vi "GIS Poll Process.vi"(8 "error in (no error)":errorcluster, 9 "notifierSync":refnum<notifier>, 10 "TopLevel":refnum<class "TopLevel.lvclass">, 11 "GIS Printer in":refnum<class "GIS Printer.lvclass">) -> (0 "error out":errorcluster, 3 "GIS Printer out":refnum<class "GIS Printer.lvclass">)   [LabVIEW 2022 SP3, in "GIS Printer.lvclass"]
uses:
  GIS Printer.lvclass
  TopLevel/TopLevel.lvclass
  GIS Printer.lvclass/GIS Printer.ctl
  Typedefs/GIS_PollTimers--cluster.ctl
  Methods/Variant_To_DVR.vi
  Methods/Generate PollStatus Event GIS Printer.vi
panel:
  in  "C1":bool
  in  "A1":bool
  in  "C2":bool
  in  "A2":bool
  in  "C3":bool
  in  "A3":bool
  in  "C4":bool
  in  "A4":bool
  in  "C33":bool
  in  "I33 3":bool
  in  "I33 2":bool
  in  "I33 1":bool
  in  "A33":bool
  in  "C22":bool
  in  "A22":bool
  in  "C11":bool
  in  "A11":bool
  in  "OK":bool
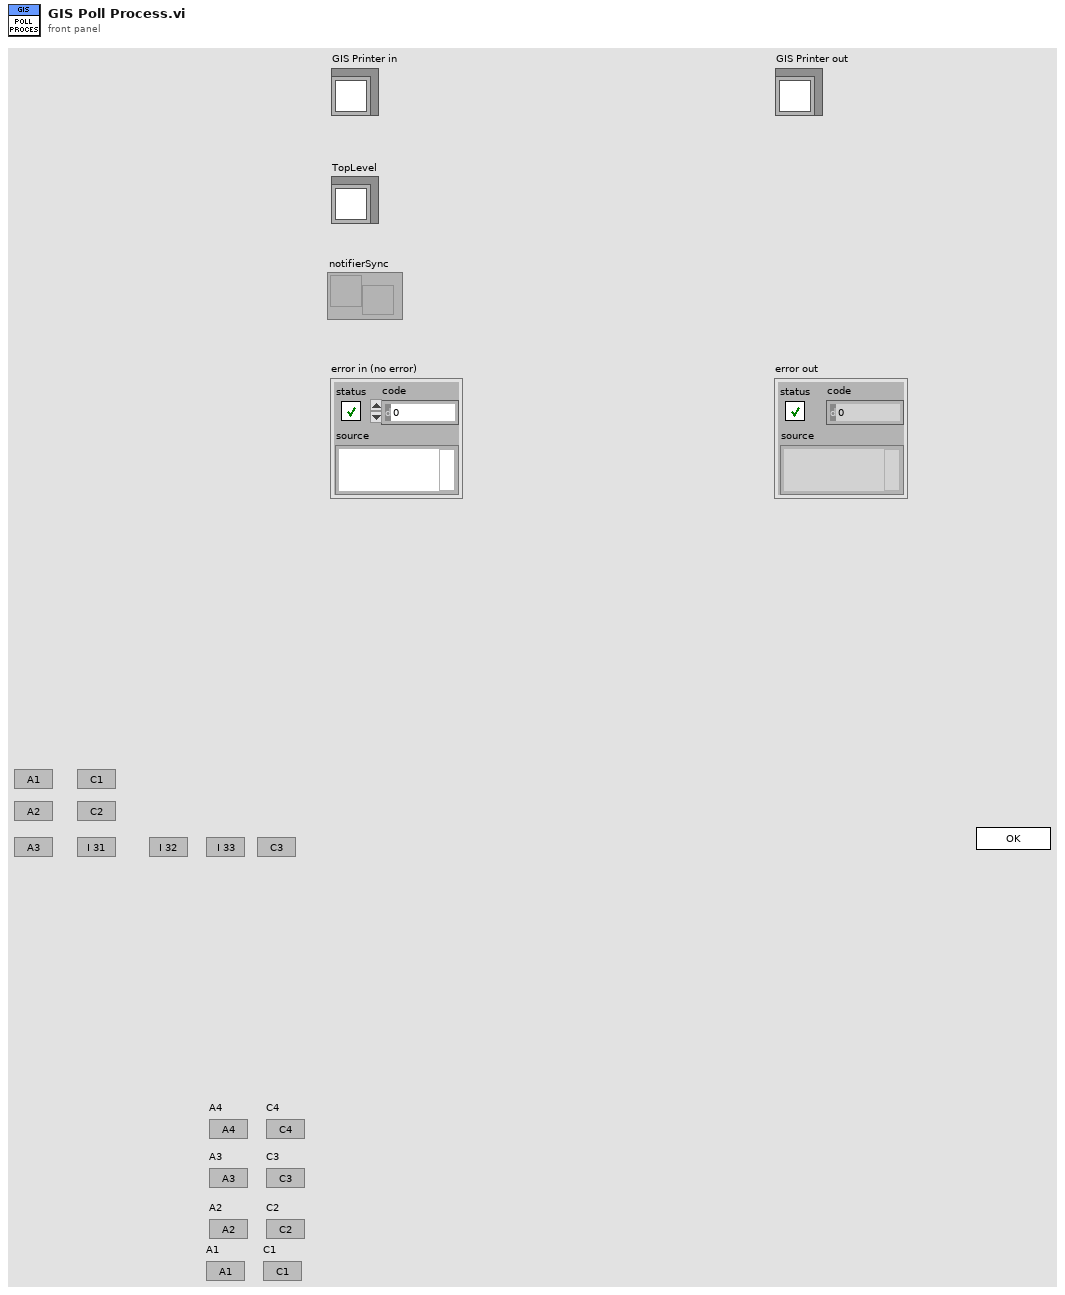
[diagram p1: front panel]
types:
  T1 = cluster{"String":string, "PrinterPollResponse":refnum<user-event>, "Open":bool, "TCP":refnum<k5>}
  T2 = enum32{"Invalid", "Standard", "Closed", "Hidden", "Minimized", "Maximized"}
  T3 = enum32{"invalid app kind", "Development System", "Run Time System", "Student Edition", "Embedded LabVIEW", "Evaluation", "Custom"}
  T4 = typedef "GIS Status--Cluster.ctl" = cluster{"HeadEnabled":bool, "SpitEnabled":bool, "HeaterEnabled":bool, "TargetTemperature":dbl, "CurrentTemperature":dbl}
  T5 = typedef "GIS Printer.lvclass/PrinterConfiguration--Cluster.ctl" = cluster{"IPAddress":string, "Move Stage on RTP Command?":bool, "Stage Move Position":string, "PH1-Prime Path":path, "PH2-Prime Path":path, "PH3-Prime Path":path, "PH4-Prime Path":path, "PH5-Prime Path":path, "PH6-Prime Path":path, "PrintScriptsFolder":path, "PurgeScriptsFolder":path, "StageScriptsFolder":path, "PH1-HeatOn Path":path, "PH2-HeatOn Path":path, "PH3-HeatOn Path":path, "PH4-HeatOn Path":path, "PH5-HeatOn Path":path, "PH6-HeatOn Path":path, "PH1-HeatOff Path":path, "PH2-HeatOff Path":path, "PH3-HeatOff Path":path, "PH4-HeatOff Path":path, "PH5-HeatOff Path":path, "PH6-HeatOff Path":path}
  T6 = typedef "GIS_PollTimers--cluster.ctl" = cluster{"HeadStatus":dbl}
  T7 = cluster{"GIS Printer in":refnum<class "GIS Printer.lvclass">, "Core":cluster{"Current VI Reference":refnum<vi>, "Close Panel on Exit?":bool}, "PrinterConfiguration":T5, "TCP":refnum<k5>, "PollTimers":T6, "PollTracker":cluster{"HeadStatusPollStart":dbl, "Poll":bool}, "notifierSync":refnum<notifier>, "PollEnable":bool}
  T8 = cluster{"Current VI Reference":refnum<vi>, "Close Panel on Exit?":bool}
  T9 = typedef "TopLevel.lvclass/Digilens Config Cluster.ctl" = cluster{"Motion Controller":T10, "IO Config":T11, "PrinterConfiguration":T5, "DAQ Settings":T14}
  T10 = typedef "Motor Controller.lvclass/Motor Controller Config Data.ctl" = cluster{"Motor IP Addresss":string, "Current Position":i32, "Pulse_Per_mm":i32, "PrePrint":dbl[], "Load Position_mm":i32, "Laminate Position_mm":i32}
  T11 = typedef "IO.lvclass/IO Config Data.ctl" = cluster{"DAQDevices":T12[], "DI Channels":T13[], "DO Channels":T13[], "Material Names":string[], "AI Channels":T13[], "AO Channels":T13[]}
  T12 = typedef "IO.lvclass/DCON_DeviceConfig--Cluster.ctl" = cluster{"COM":string, "DeviceName":string, "BaudRate":u32, "Number of Channels":i32, "DeviceAddress":i32, "Enable":bool}
  T13 = typedef "IO.lvclass/Channel Data.ctl" = cluster{"Channel Name":string, "Device Name":string, "Channel No":string}
  T14 = typedef "DAQ.lvclass/TD DAQ Settings--cluster.ctl" = cluster{"Simulate DAQ":bool, "DI Settings":T15[], "AI Settings":T16[], "Relay IONames":string[], "AO IONames":string[], "AO NChan SingleTask":bool}
  T15 = typedef "DAQ.lvclass/TD DI Instrument Settings--cluster.ctl" = cluster{"Disable":bool, "DI TaskName":string, "DI RefreshIntv":i32}
  T16 = typedef "DAQ.lvclass/TD AI Instrument Settings--cluster.ctl" = cluster{"Disable":bool, "AI TaskName":string, "AI InstSettings":T17, "SimAI Ranges":T18}
  T17 = typedef "DAQ.lvclass/TD AI InstSettings--cluster.ctl" = cluster{"DaqRate":dbl, "NumSamples":i32}
  T18 = typedef "DAQ.lvclass/TD SimAI Ranges--cluster.ctl" = cluster{"lo":dbl, "hi":dbl}
  T19 = typedef "TopLevel.lvclass/UserEvents.ctl" = cluster{"API Incoming Event":refnum<user-event>, "API Executed Event":refnum<user-event>, "API Return Event":refnum<user-event>, "Exit Event":refnum<user-event>, "StatusChanged":refnum<user-event>, "DLP GUI Config Changed":refnum<user-event>, "AppEvent":refnum<user-event>, "Login Event":refnum<user-event>}
  T20 = typedef "GIS Printer.lvclass/UserEvents.ctl" = cluster{"API Incoming Event":refnum<user-event>, "API Executed Event":refnum<user-event>, "API Return Event":refnum<user-event>, "Status Changed Event":refnum<user-event>, "Abort":refnum<user-event>, "stop process":refnum<user-event>, "GISPollStatus":refnum<user-event>, "GISHeadStatus":refnum<user-event>, "Error Event":refnum<user-event>}
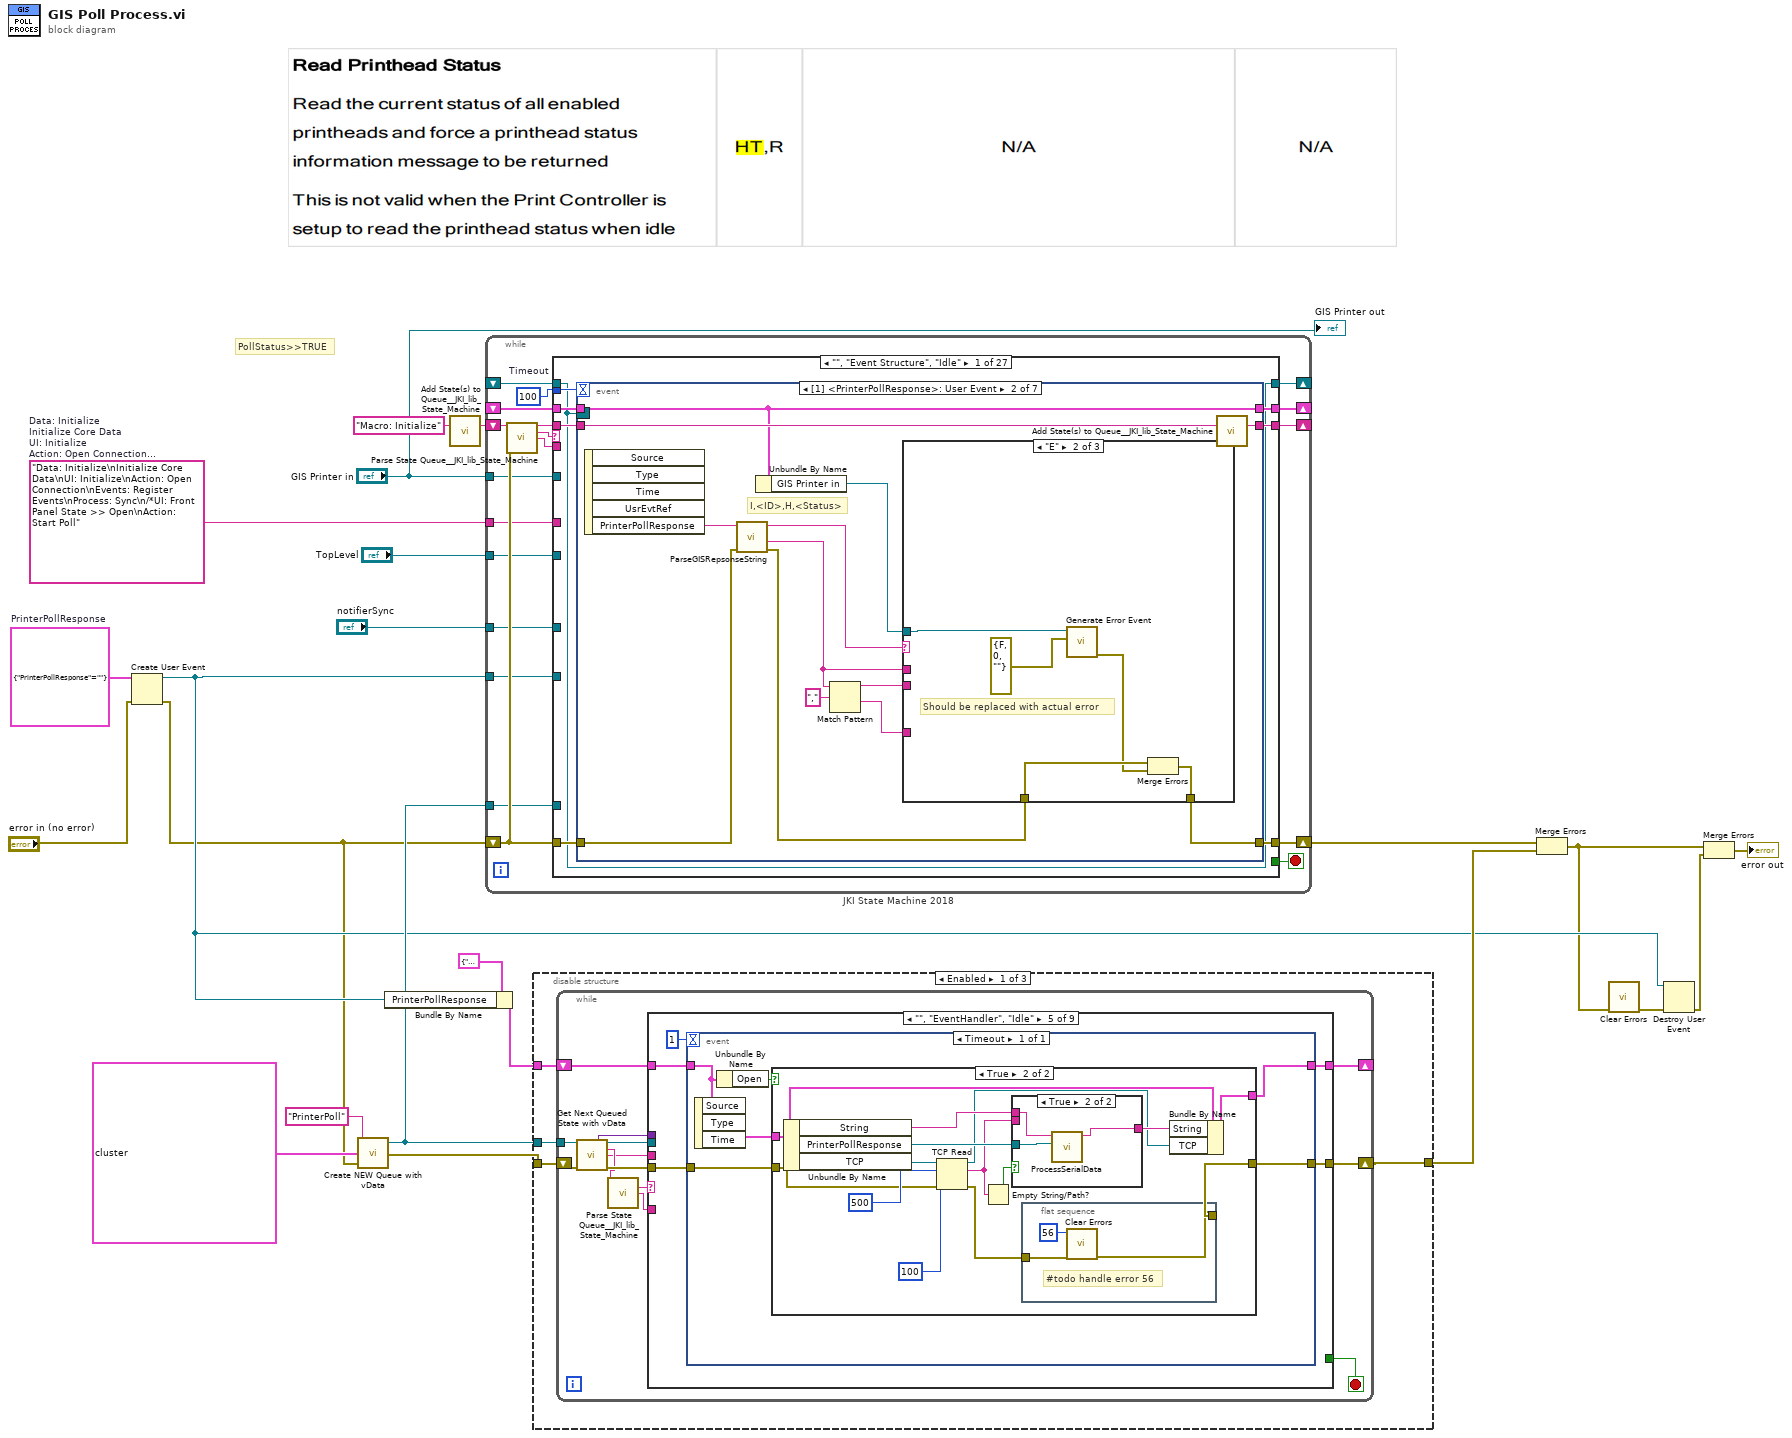
[diagram p0: block diagram]
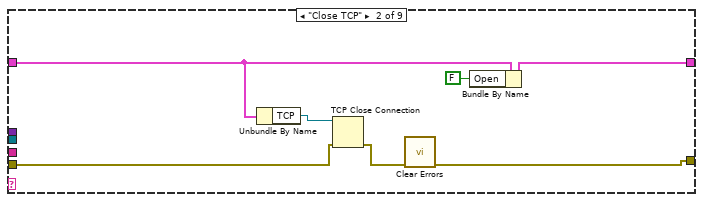
[diagram p3: hidden frame]
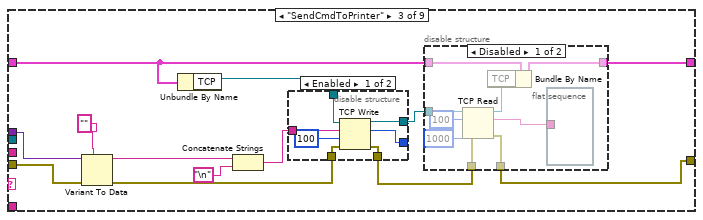
[diagram p4: hidden frame]
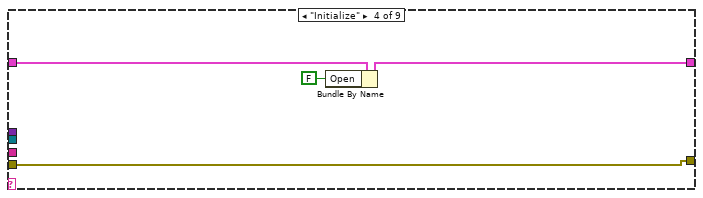
[diagram p7: hidden frame]
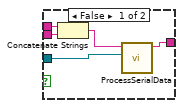
[diagram p9: hidden frame]
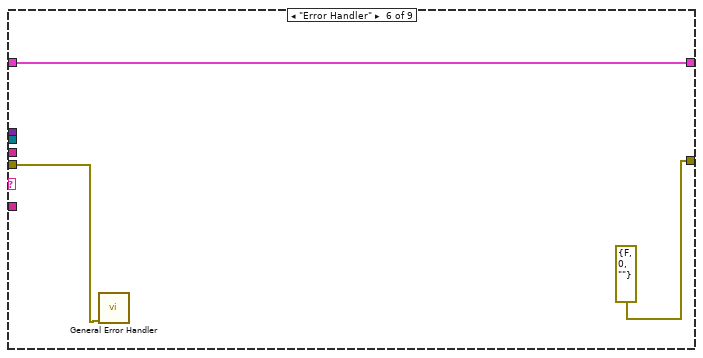
[diagram p10: hidden frame]
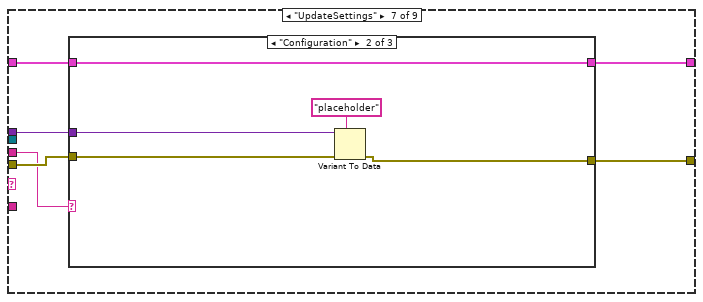
[diagram p11: hidden frame]
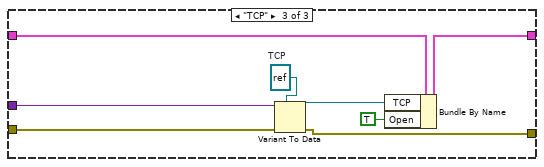
[diagram p13: hidden frame]
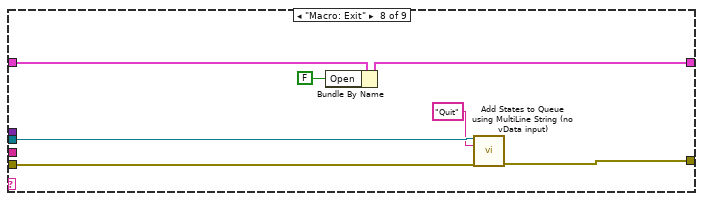
[diagram p14: hidden frame]
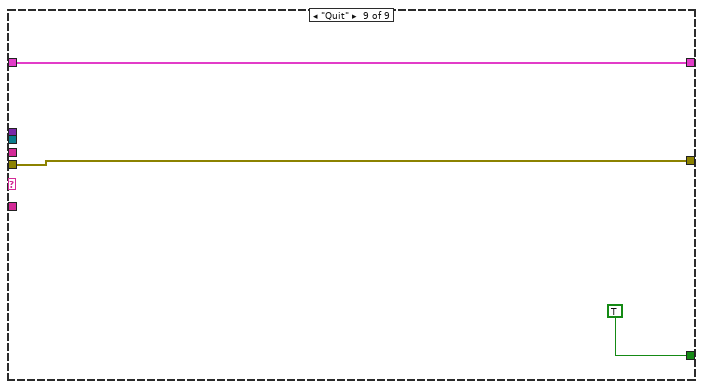
[diagram p15: hidden frame]
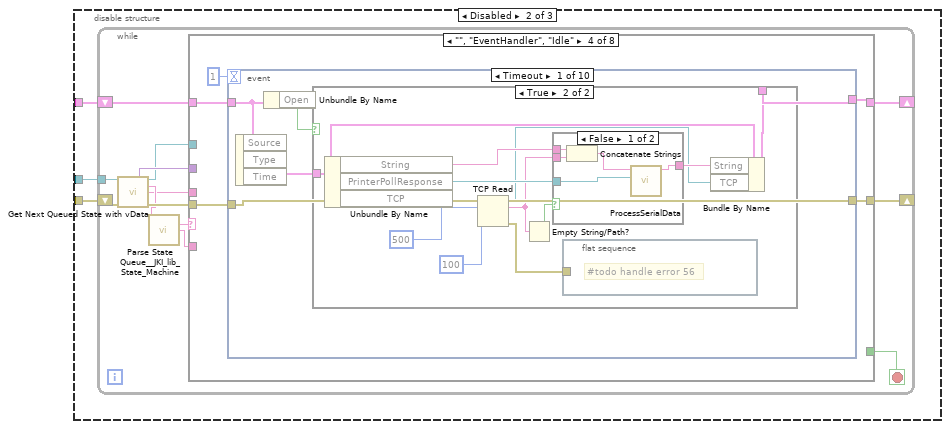
[diagram p16: hidden frame]
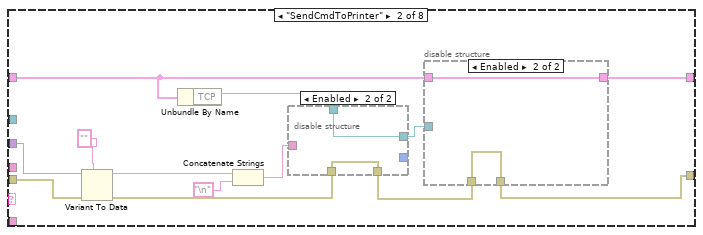
[diagram p18: hidden frame]
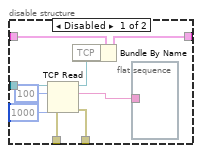
[diagram p19: hidden frame]
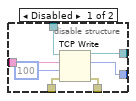
[diagram p20: hidden frame]
diagram:
  w1 = "Data: Initialize\nInitialize Core Data\nUI: Initialize\nAction: Open Connection\nEvents: Register Events\nProcess: Sync\n/*UI: Front Panel State >> Open\nAction: Start Poll"  # Data: Initialize Initialize Core Data UI: Initialize Action: Open Connection Events: Register Events Process: Sync /*UI: Front Panel State >> Open Action: Start Poll
  w13 = cluster{"PrinterPollResponse":string} {"PrinterPollResponse"=""}  # PrinterPollResponse
  # "PollStatus>>TRUE"
  n1 = Create User Event(user event datatype=w13, error in="error in (no error)") -> (user event=w10:refnum<user-event>, error out=w2:errorcluster)
  n2 = call <vilib>:"Create NEW Queue with vData.vi"("error in (no error)"=w2, "Initial States"=cluster{"state":string, "vData":variant}[] [{"state"="Initialize", "vData"=variant}, {"state"="Idle", "vData"=variant}], "Name (SMQ)"="PrinterPoll") -> ("error out"=w18:errorcluster, "queue out"=w14:refnum<queue>)  [unwired: 1 in]
  n3 = Bundle By Name(cluster=T1 {"String"="", "PrinterPollResponse"=refnum, "Open"=FALSE, "TCP"=refnum}, "PrinterPollResponse"=w10) -> (w15:T1)
  n4 = call <vilib>:"Add State(s) to Queue__JKI_lib_State_Machine.vi"("State(s) in (\"\")"="Macro: Initialize") -> ("States Out"=w22:string)  [unwired: 14 in]
  n5 = while "JKI State Machine 2018" {
    shift-right: [w34] -> _
    shift-left: _ -> [w33]
    shift-right: [w37] -> w12
    shift-left: w2 -> [w31]
    shift-right: [w36] -> _
    shift-left: w22 -> [w38]
    tunnel: "GIS Printer in" -> [w30]
    tunnel: "TopLevel" -> [w29]
    tunnel: w14 -> [w28]
    tunnel: w10 -> [w27]
    shift-right: [w26] -> _
    shift-left: _ -> [w25]
    tunnel: "notifierSync" -> [w24]
    tunnel: w1 -> [w23]
    stop <- w35 stop-if-true
    w32 = 100  # Timeout
    n6 = call <vilib>:"Parse State Queue__JKI_lib_State_Machine.vi"("State Queue"=w38, "Error In (no error)"=w31) -> ("Remaining States"=w40:string, "Current State"=w41:string, "Arguments"=w39:string)  [unwired: 11 in]
    n7 = case shown="\"\", \"Event Structure\", \"Idle\"" w41 {
      selector: w41 -> [_ _ w136 _ _ _ _ _ _ _ _ _ _ _ _ _ _ _ _ _ _ _ _ _ _ _ _]
      tunnel: w40 -> [w49 w134 w140 w160 w167 w176 w181 w188 w202 w217 w224 w229 w234 w241 w253 w323 w329 w340 w345 w353 w361 w375 w384 w399 w405 w417 w428]
      tunnel: w39 -> [_ _ _ _ _ _ _ _ _ _ _ _ _ w236 w247 _ _ _ _ _ _ _ _ _ _ w413 _]
      tunnel: w33 -> [w47 w131 w138 w153 w164 w174 w178 w186 w195 _ w219 w226 w232 w239 w249 w320 w326 w337 w342 w350 w356 w371 w381 w394 w403 w415 w418]
      tunnel: [w46 w132 w142 w157 errorcluster {"status"=FALSE, "code"=0, "source"=""} ("error out") w169 w179 w184 w191 w203 w220 w227 w231 w237 w250 w321 w327 w338 w343 w347 w355 w373 w382 w390 w401 w411 w421] -> w37
      tunnel: w31 -> [w45 w132 w141 w157 w163 w168 w179 w183 w197 w203 w221 w227 w231 w238 w251 w321 w327 w338 w343 w346 w354 w373 w382 w386 w400 w410 w420]
      tunnel: [w48 w133 w139 w159 w166 w175 w180 w187 w201 w216 w223 w228 w233 w240 w252 w322 w328 w339 w344 w352 w360 w374 w383 w398 w404 w416 w427] -> w36
      tunnel: [_ _ _ _ _ TRUE _ _ _ _ _ _ _ _ _ _ _ _ _ _ _ _ _ _ _ _ _] -> w35
      tunnel: [w44 w131 w138 w158 w164 w174 w178 w186 w196 w215 w219 w226 w232 w239 w249 w320 w326 w337 w342 w350 w356 w371 w379 w394 w403 w408 w419] -> w34
      tunnel: w32 -> [w43 _ _ _ _ _ _ _ _ _ _ _ _ _ _ _ _ _ _ _ _ _ _ _ _ _ _]
      tunnel: w30 -> [_ _ _ _ _ _ _ _ _ w204 _ _ _ _ _ _ _ _ _ _ _ _ _ _ _ _ _]
      tunnel: w29 -> [_ _ _ _ _ _ _ _ _ w213 _ _ _ _ _ _ _ _ _ _ _ _ _ w388 _ _ _]
      tunnel: w28 -> [_ _ _ _ _ w170 _ _ w193 _ _ _ _ _ _ _ _ _ _ w348 _ _ _ _ _ w412 w422]
      tunnel: w27 -> [_ _ _ _ _ _ _ _ _ _ _ _ _ _ _ _ _ _ _ _ _ _ _ w397 _ _ _]
      tunnel: [w42 w130 w135 w147 w161 w172 w177 w182 w189 w209 w218 w225 w230 w235 w246 w319 w325 w330 w341 w351 w359 w372 w380 w396 w402 w409 w426] -> w26
      tunnel: w25 -> [w42 w130 w135 w147 w161 w172 w177 w182 w189 w209 w218 w225 w230 w235 w246 w319 w325 w330 w341 w351 w359 w372 w380 _ w402 w409 w426]
      tunnel: w24 -> [_ _ _ _ _ _ _ _ _ w206 _ _ _ _ _ _ _ _ _ _ _ _ _ _ _ _ _]
      tunnel: w23 -> [_ _ _ _ _ _ _ _ _ _ _ _ _ _ _ _ w324 _ _ _ _ _ _ _ _ _ _]
      frame "", "Event Structure", "Idle" {
        n8 = event shown="[1] <PrinterPollResponse>: User Event" {
          selector: w42 -> [_ _ _ _ _ _ _]
          dyn-events: _ -> [_ _ _ _ _ _ _]
          timeout: w43 -> [_ _ _ _ _ _ _]
          tunnel: w49 -> [w57 w71 w97 w102 w106 w114 w129]
          tunnel: [w56 w70 w96 w101 w105 w113 w128] -> w48
          tunnel: w47 -> [w53 w63 w94 w99 w103 w109 w126]
          tunnel: [w55 w61 w95 w100 w104 w108 w127] -> w46
          tunnel: w45 -> [w55 w59 w95 w100 w104 w107 w127]
          tunnel: [w53 w63 w94 w99 w103 w110 w126] -> w44
          event Timeout {
            n9 = event-data() -> ()  [unwired: 1 in, 1 out]
            n10 = Unbundle By Name(w53) -> ("PollTracker.Poll"=w52:bool, "PollEnable"=w50:bool)
            n11 = And(x=w52, y=w50) -> (x .and. y?=w51:bool)
            n12 = case shown="True" w51 {
              tunnel: [_ "Action: CheckPollTimers" ("State(s) in Front (\"\")")] -> w54
              frame False {
              }
              frame True {
              }
            }
            n13 = call <vilib>:"Add State(s) to Queue__JKI_lib_State_Machine.vi"("State(s) in Front (\"\")"=w54, "State(s) in (\"\")"=w57) -> ("States Out"=w56:string)  [unwired: 13 in]
          }
          event User Event {
            # "I,<ID>,H,<Status>"
            n14 = event-data() -> ("PrinterPollResponse"=w69:string)  [unwired: 1 in, 4 out]
            n15 = call "ParseGISRepsonseString.vi"("error in (no error)"=w59, "Response In"=w69) -> ("error out"=w60:errorcluster, "Status"=w66:string, "Category"=w68:string)  [unwired: 6 in, 1 out]
            n16 = Unbundle By Name(w63) -> ("GIS Printer in"=w62:refnum<class "GIS Printer.lvclass">)
            n17 = Match Pattern(string=w66, regular expression=",") -> (before substring=w65:string, after substring=w64:string)  [unwired: 1 in, 2 out]
            n18 = case shown="\"E\"" w68 {
              tunnel: w66 -> [_ _ _]
              tunnel: w65 -> [_ _ w84]
              tunnel: w64 -> [_ _ w81]
              tunnel: w62 -> [_ w77 w80]
              tunnel: w60 -> [w72 w75 w79]
              tunnel: [w72 w73 w78] -> w61
              frame Default {
              }
              frame "E" {
                # "Should be replaced with actual error"
                n19 = call-dynamic "Generate Error Event.vi"("Error"=errorcluster {"status"=FALSE, "code"=0, "source"=""}, "GIS Printer in"=w77) -> ("error out"=w74:errorcluster)  [unwired: 8 in, 1 out]
                n20 = Merge Errors(w75, w74) -> (w73:errorcluster)
              }
              frame "I" {
                n21 = Equal?(x=w84, y="H") -> (x = y?=w82:bool)
                n22 = case shown="True" w82 {
                  tunnel: w81 -> [_ w92]
                  tunnel: w80 -> [_ w90]
                  tunnel: w79 -> [w85 w91]
                  tunnel: [w85 w87] -> w78
                  frame False {
                  }
                  frame True {
                    n23 = call "GISStatus_XML_Read.vi"("error in (no error)"=w91, "XML String"=w92) -> ("error out"=w88:errorcluster, "HeadStatus"=w89:T4[])  [unwired: 7 in, 1 out]
                    n24 = call "Write GISPollStatus.vi"("ForceEvent"=TRUE, "error in (no error)"=w88, "GISHeadStatus"=w89, "GIS Printer in"=w90) -> ("error out"=w87:errorcluster)  [unwired: 6 in, 1 out]
                  }
                }
              }
            }
            n25 = call <vilib>:"Add State(s) to Queue__JKI_lib_State_Machine.vi"("State(s) in (\"\")"=w71) -> ("States Out"=w70:string)  [unwired: 14 in]
          }
          event "OK": Value Change {
            # "Exit Button Value Change (pressed) Event\n(this executes Macro: Exit to terminate the VI)"
            n26 = event-data() -> ()  [unwired: 1 in, 1 out]
            n27 = call <vilib>:"Add State(s) to Queue__JKI_lib_State_Machine.vi"("State(s) in Front (\"\")"="Macro: Exit", "State(s) in (\"\")"=w97) -> ("States Out"=w96:string)  [unwired: 13 in]
          }
          event User Event {
            # "Exit Button Value Change (pressed) Event\n(this executes Macro: Exit to terminate the VI)"
            n28 = event-data() -> ()  [unwired: 1 in, 5 out]
            n29 = call <vilib>:"Add State(s) to Queue__JKI_lib_State_Machine.vi"("State(s) in Front (\"\")"="Macro: Exit", "State(s) in (\"\")"=w102) -> ("States Out"=w101:string)  [unwired: 13 in]
          }
          event User Event {
            # "#TODO API: Abort called in  other process. do something about it man!\njust do something...anything"
            # "Exit Button Value Change (pressed) Event\n(this executes Macro: Exit to terminate the VI)"
            n30 = event-data() -> ()  [unwired: 1 in, 5 out]
            n31 = call <vilib>:"Add State(s) to Queue__JKI_lib_State_Machine.vi"("State(s) in (\"\")"=w106) -> ("States Out"=w105:string)  [unwired: 14 in]
          }
          event User Event {
            n32 = event-data() -> ("Command"=w112:string, "Data"=w111:variant)  [unwired: 1 in, 4 out]
            n33 = case shown="\"StatusPoll\"" w112 {
              tunnel: w111 -> [_ w123]
              tunnel: w109 -> [w116 w121]
              tunnel: [w116 w120] -> w110
              tunnel: w107 -> [w115 w118]
              tunnel: [w115 w117] -> w108
              frame Default {
              }
              frame "StatusPoll" {
                n34 = Variant To Data(error in=w118, type=FALSE, Variant=w123) -> (data=w119:bool, error out=w117:errorcluster)
                n35 = Bundle By Name(cluster=w121, "PollEnable"=w119) -> (w120:T7)
              }
            }
            n36 = call <vilib>:"Add State(s) to Queue__JKI_lib_State_Machine.vi"("State(s) in (\"\")"=w114) -> ("States Out"=w113:string)  [unwired: 14 in]
          }
          event Panel Close? {
            # "Discard the event because we'll close the front panel ourselves in Macro: Exit"
            # "Close Panel button (pressed) Event\n(this executes Macro: Exit to terminate the VI)"
            n37 = event-data() -> ()  [unwired: 1 in, 1 out]
            n38 = event-data("Discard?"=TRUE) -> ()  [unwired: 1 in, 1 out]
            n39 = call <vilib>:"Add State(s) to Queue__JKI_lib_State_Machine.vi"("State(s) in Front (\"\")"="Macro: Exit", "State(s) in (\"\")"=w129) -> ("States Out"=w128:string)  [unwired: 13 in]
          }
        }
      }
      frame "---------- Core ----------" {
        # "Do not put any code in this frame.\n(it is a separator no-op)"
        n40 = call <vilib>:"Add State(s) to Queue__JKI_lib_State_Machine.vi"("State(s) in (\"\")"=w134) -> ("States Out"=w133:string)  [unwired: 14 in]
      }
      frame Default {
        w145 = 42 items=["No error", "Argument error", "Memory is full", "Out of zone", "End of file", "File already open", "Generic file I/O error", "File not found", "File permission error", "Disk is full", "Duplicate path", "Too many files open", "System feature not enabled", "Resource file not found", "Cannot add resource", "Resource not found", "Image not found", "Image memory error", "Pen does not exist", "Config type invalid", "Config token not found", "Config parse error", "Config memory error", "Bad external code format", "Bad external code offset", "External code not present", "Null window", "Destroy window error", "Null menu", "Print aborted", "Bad print record", "Print driver error", "Windows error during printing", "Memory error during printing", "Print dialog error", "Generic print error", "Invalid device refnum", "Device not found", "Device parameter error", "Device unit error", "Cannot open device", "Device call aborted", "Generic error", "Cancelled by user", "Object ID too low", "Object ID too high", "Object not in heap", "Unknown heap", "Unknown object (invalid DefProc)", "Unknown object (DefProc not in table)", "Message out of range", "Invalid (null) method", "Unknown message", "Manager call not supported", "Bad address", "Network operation in progress", "Network operation timed out", "Connection is busy", "Network attribute not supported", "Network error", "Address in use", "System out of memory", "Connection aborted", "Connection refused", "Not connected", "Already connected", "Connection closed", "Initialization error (interapplication manager)", "Bad occurrence", "Wait on unbound occurrence handler", "Occurrence queue overflow", "Datalog type conflict", "Unused", "Unrecognized type (interapplication manager)", "Memory corrupt", "Failed to make temporary DLL", "Old CIN version", "Drag socket not found", "Failed to load drop-object", "Failed to register OLE object", "Failed to release OLE object", "Format specifier type mismatch", "Unknown format specifier", "Too few format specifiers", "Too many format specifiers", "Scan failed", "Newer CIN version", "Error converting to variant", "Runtime menu error", "Password tampered", "Variant attribute not found", "Incompatible variant data type", "Event data is not available", "Event Store is not present", "Occurrence is not found", "Event Queue is not created", "Event info is not available", "Refnum passed is NULL", "Error retrieving Class GUID", "Error retrieving CoClass GUID", "Error retrieving TypeLib GUID.", "Bad built application magic bytes.", "Specific driver is different from the specific driver associated with the Logical Name.", "There is no session opened to the class driver.", "Max Error", "MAX - Error with config objects", "MAX - Error loading configuration", "MAX - Group not supported"]
        # "Current State"
        # "Do not delete, rename, or modify this frame.\n(this is used to capture unhandled states and typos)"
        # "Handle mistyped state name (developer tool)"
        n41 = Format Into String(format string="Software Exception: Unhandled State \"%s\"." ("message"), error in=w141, w136) -> (resulting string=w144:string, error out=w143:errorcluster)  [unwired: 1 in]
        n42 = call <vilib>:"Error Cluster From Error Code.vi"("show call chain? (False)"=TRUE, "error in (no error)"=w143, "error message (\"\")"=w144, "error code (0)"=w145) -> ("error out"=w142:errorcluster)  [unwired: 5 in]
        n43 = call <vilib>:"Add State(s) to Queue__JKI_lib_State_Machine.vi"("State(s) in (\"\")"=w140) -> ("States Out"=w139:string)  [unwired: 14 in]
      }
      frame "Initialize Core Data" {
        # "Do not delete, rename, or modify this frame.\n(this is used to determine panel behavior on exit)"
        # "originally closed?"
        # "exe?"
        # "If panel starts closed or is an EXE, then close it when we exit"
        n44 = property class="VI"() -> ("FP.State"=w150:T2)  [unwired: 2 in, 2 out]
        n45 = property class="App"() -> ("App.Kind"=w156:T3)  [unwired: 2 in, 2 out]
        n46 = control-ref of="Current VI Reference"() -> (w151:refnum<vi>)
        n47 = Equal?(x=w150, y=T2."Closed" ("Front Panel Window:State")) -> (x = y?=w148:bool)
        n48 = Equal?(x=w156, y=T3."Run Time System" ("Application:Kind")) -> (x = y?=w154:bool)
        n49 = Or(x=w148, y=w154) -> (x .or. y?=w152:bool)
        n50 = Bundle By Name(cluster=w153, "Core.Current VI Reference"=w151, "Core.Close Panel on Exit?"=w152) -> (w158:T7)
        n51 = call <vilib>:"Add State(s) to Queue__JKI_lib_State_Machine.vi"("State(s) in (\"\")"=w160) -> ("States Out"=w159:string)  [unwired: 14 in]
      }
      frame "Error Handler" {
        # "Unhandled Error -- Display it"
        # "Handle any errors here.\nYou can also output any states to clean-up after errors occur"
        # "Clear error"
        n52 = call <vilib>:"General Error Handler.vi"("error in (no error)"=w163) -> ()  [unwired: 10 in, 5 out]
        n53 = call <vilib>:"Add State(s) to Queue__JKI_lib_State_Machine.vi"("State(s) in Front (\"\")"="/* Post Error States", "State(s) in (\"\")"=w167) -> ("States Out"=w166:string)  [unwired: 13 in]
      }
      frame "Exit" {
        n54 = call <vilib>:"Add States to Queue using MultiLine String (no vData input).vi"("queue in"=w170, "states in"="Quit", "error in"=w168) -> ("error out"=w169:errorcluster)  [unwired: 10 in, 2 out]
        n55 = call <vilib>:"Add State(s) to Queue__JKI_lib_State_Machine.vi"("State(s) in (\"\")"=w176) -> ("States Out"=w175:string)  [unwired: 14 in]
      }
      frame "---------- Data ----------" {
        # "Do not put any code in this frame.\n(It is a separator no-op. You can make a copy of this frame to create a new Data frame)"
        n56 = call <vilib>:"Add State(s) to Queue__JKI_lib_State_Machine.vi"("State(s) in (\"\")"=w181) -> ("States Out"=w180:string)  [unwired: 14 in]
      }
      frame "Data: GIS Disconnect" {
        # "Do not put any code in this frame.\n(It is a separator no-op. You can make a copy of this frame to create a new Data frame)"
        n57 = Unbundle By Name(w186) -> ("TCP"=w185:refnum<k5>)
        n58 = TCP Close Connection(connection ID=w185, error in (no error)=w183) -> (error out=w184:errorcluster)  [unwired: 1 in, 1 out]
        n59 = call <vilib>:"Add State(s) to Queue__JKI_lib_State_Machine.vi"("State(s) in (\"\")"=w188) -> ("States Out"=w187:string)  [unwired: 14 in]
      }
      frame "Data: GIS Connect" {
        n60 = Unbundle By Name(w195) -> ("PrinterConfiguration.IPAddress"=w200:string)
        n61 = TCP Open Connection(address=w200, remote port or service name=u16 2000, timeout ms (60000)=1000, error in (no error)=w197) -> (connection ID=w190:refnum<k5>, error out=w192:errorcluster)  [unwired: 1 in]
        n62 = call <vilib>:"Add State to Queue with vData.vi"("queue in"=w193, "state in"="UpdateSettings>>TCP", "vData (\"\")"=w190, "error in"=w192) -> ("error out"=w191:errorcluster)  [unwired: 8 in, 3 out]
        n63 = Bundle By Name(cluster=w195, "TCP"=w190) -> (w196:T7)
        n64 = call <vilib>:"Add State(s) to Queue__JKI_lib_State_Machine.vi"("State(s) in (\"\")"=w202) -> ("States Out"=w201:string)  [unwired: 14 in]
      }
      frame "Data: Initialize" {
        w205 = TRUE  # PollEnable
        w207 = cluster{"HeadStatusPollStart":dbl, "Poll":bool} {"HeadStatusPollStart"=0.0, "Poll"=FALSE}  # PollTracker
        w208 = T6 {"HeadStatus"=2.0}  # PollTimers
        w210 = refnum<k5> refnum  # TCP
        w214 = T8 {"Current VI Reference"=refnum, "Close Panel on Exit?"=FALSE}  # Core
        # "#TODO get from config"
        n65 = property class="TopLevel.lvclass"(reference=w213) -> ("Methods:Accessors:Digilens Config"=w212:T9)  [unwired: 1 in, 2 out]
        n66 = Unbundle By Name(w212) -> ("PrinterConfiguration"=w211:T5)
        n67 = Bundle("GIS Printer in"=w204, "Core"=w214, "PrinterConfiguration"=w211, "TCP"=w210, "PollTimers"=w208, "PollTracker"=w207, "notifierSync"=w206, "PollEnable"=w205) -> (w215:T7)  [unwired: 1 in]
        n68 = call <vilib>:"Add State(s) to Queue__JKI_lib_State_Machine.vi"("State(s) in (\"\")"=w217) -> ("States Out"=w216:string)  [unwired: 14 in]
      }
      frame "Data: Cleanup" {
        # "Cleanup any data and references, here.\n(this is called automatically, by the Macro: Exit)"
        n69 = Unbundle By Name(w219) -> ("Core.Current VI Reference"=w222:refnum<vi>)
        n70 = Close Reference(reference=w222, error in (no error)=w221) -> (error out=w220:errorcluster)
        n71 = call <vilib>:"Add State(s) to Queue__JKI_lib_State_Machine.vi"("State(s) in (\"\")"=w224) -> ("States Out"=w223:string)  [unwired: 14 in]
      }
      frame "---------- UI ----------" {
        # "Do not put any code in this frame.\n(It is a separator no-op. You can make a copy of this frame to create a new UI frame)"
        n72 = call <vilib>:"Add State(s) to Queue__JKI_lib_State_Machine.vi"("State(s) in (\"\")"=w229) -> ("States Out"=w228:string)  [unwired: 14 in]
      }
      frame "UI: Initialize" {
        n73 = call <vilib>:"Add State(s) to Queue__JKI_lib_State_Machine.vi"("State(s) in (\"\")"=w234) -> ("States Out"=w233:string)  [unwired: 14 in]
      }
      frame "UI: Cursor Set" {
        # "Argument"
        # "Set and Unset Cursor Busy.\n(Usage: \"UI: Cursor Set >> Busy|Idle\")"
        n74 = case shown="\"Idle\", Default" w236 {
          tunnel: w238 -> [w243 w245]
          tunnel: [w242 w244] -> w237
          frame "Idle", Default {
            n75 = call <vilib>:"Unset Busy.vi"("error in (no error)"=w243) -> ("error out"=w242:errorcluster)  [unwired: 10 in]
          }
          frame "Busy" {
            n76 = call <vilib>:"Set Busy.vi"("error in (no error)"=w245) -> ("error out"=w244:errorcluster)  [unwired: 9 in, 1 out]
          }
        }
        n77 = call <vilib>:"Add State(s) to Queue__JKI_lib_State_Machine.vi"("State(s) in (\"\")"=w241) -> ("States Out"=w240:string)  [unwired: 14 in]
      }
      frame "UI: Front Panel State" {
        # "Argument"
        # "Set Front Panel Open or Closed\n(Usage: \"UI: Front Panel State >> Open|Close\")"
        n78 = Unbundle By Name(w249) -> ("Core.Current VI Reference"=w248:refnum<vi>)
        n79 = case shown="\"Minimize\", \"Minimized\"" w247 {
          tunnel: w251 -> [w259 w274 w285 w298 w311]
          tunnel: [w261 w275 w287 w300 w313] -> w250
          tunnel: w248 -> [w260 w272 w286 w299 w312]
          frame "Open", "Standard", Default {
            w254 = T2."Standard" ("State")
            n80 = property class="VI"(reference=w260, error in=w259) -> (reference out=w257:refnum<vi>, error out=w258:errorcluster, "FP.State"=w256:T2)
            n81 = Not Equal?(x=w256, y=w254) -> (x != y?=w255:bool)
            n82 = case shown="True" w255 {
              tunnel: [w265 w267] -> w261
              tunnel: w258 -> [w264 w267]
              tunnel: w257 -> [w263 _]
              tunnel: w254 -> [w262 _]
              frame True {
                n83 = invoke class="VI" method="FP.Open"(reference=w263, error in=w264, "Activate"=TRUE, "State"=w262) -> (error out=w265:errorcluster)  [unwired: 1 in, 4 out]
              }
              frame False {
              }
            }
          }
          frame "Close", "Closed" {
            n84 = property class="VI"(reference=w272, error in=w274) -> (reference out=w271:refnum<vi>, error out=w273:errorcluster, "FP.State"=w269:T2)
            n85 = Not Equal?(x=w269, y=T2."Closed" ("Front Panel Window:State")) -> (x != y?=w268:bool)
            n86 = case shown="True" w268 {
              tunnel: [w276 w279] -> w275
              tunnel: w273 -> [w276 w278]
              tunnel: w271 -> [_ w277]
              frame False {
              }
              frame True {
                n87 = invoke class="VI" method="FP.Close"(reference=w277, error in=w278) -> (error out=w279:errorcluster)  [unwired: 1 in, 2 out]
              }
            }
          }
          frame "Hidden", "Hide" {
            w280 = T2."Hidden" ("State")
            n88 = property class="VI"(reference=w286, error in=w285) -> (reference out=w283:refnum<vi>, error out=w284:errorcluster, "FP.State"=w282:T2)
            n89 = Not Equal?(x=w282, y=w280) -> (x != y?=w281:bool)
            n90 = case shown="True" w281 {
              tunnel: [w291 w292] -> w287
              tunnel: w284 -> [w290 w292]
              tunnel: w283 -> [w289 _]
              tunnel: w280 -> [w288 _]
              frame True {
                n91 = invoke class="VI" method="FP.Open"(reference=w289, error in=w290, "State"=w288) -> (error out=w291:errorcluster)  [unwired: 2 in, 4 out]
              }
              frame False {
              }
            }
          }
          frame "Minimize", "Minimized" {
            w293 = T2."Minimized" ("State")
            n92 = property class="VI"(reference=w299, error in=w298) -> (reference out=w296:refnum<vi>, error out=w297:errorcluster, "FP.State"=w295:T2)
            n93 = Not Equal?(x=w295, y=w293) -> (x != y?=w294:bool)
            n94 = case shown="True" w294 {
              tunnel: [w304 w305] -> w300
              tunnel: w297 -> [w303 w305]
              tunnel: w296 -> [w302 _]
              tunnel: w293 -> [w301 _]
              frame True {
                n95 = invoke class="VI" method="FP.Open"(reference=w302, error in=w303, "State"=w301) -> (error out=w304:errorcluster)  [unwired: 2 in, 4 out]
              }
              frame False {
              }
            }
          }
          frame "Maximize", "Maximized" {
            w306 = T2."Maximized" ("State")
            n96 = property class="VI"(reference=w312, error in=w311) -> (reference out=w309:refnum<vi>, error out=w310:errorcluster, "FP.State"=w308:T2)
            n97 = Not Equal?(x=w308, y=w306) -> (x != y?=w307:bool)
            n98 = case shown="True" w307 {
              tunnel: [w317 w318] -> w313
              tunnel: w310 -> [w316 w318]
              tunnel: w309 -> [w315 _]
              tunnel: w306 -> [w314 _]
              frame True {
                n99 = invoke class="VI" method="FP.Open"(reference=w315, error in=w316, "State"=w314) -> (error out=w317:errorcluster)  [unwired: 2 in, 4 out]
              }
              frame False {
              }
            }
          }
        }
        n100 = call <vilib>:"Add State(s) to Queue__JKI_lib_State_Machine.vi"("State(s) in (\"\")"=w253) -> ("States Out"=w252:string)  [unwired: 14 in]
      }
      frame "---------- Macro ----------" {
        # "Do not put any code in this frame.\n(It is a separator no-op. You can make a copy of this frame to create a new Macro frame)"
        n101 = call <vilib>:"Add State(s) to Queue__JKI_lib_State_Machine.vi"("State(s) in (\"\")"=w323) -> ("States Out"=w322:string)  [unwired: 14 in]
      }
      frame "Macro: Initialize" {
        n102 = call <vilib>:"Add State(s) to Queue__JKI_lib_State_Machine.vi"("State(s) in Front (\"\")"=w324, "State(s) in (\"\")"=w329) -> ("States Out"=w328:string)  [unwired: 13 in]
      }
      frame "Macro: Exit" {
        n103 = Unbundle By Name(w337) -> ("Core.Close Panel on Exit?"=w336:bool)
        n104 = Select(t="UI: Front Panel State >> Close", s=w336, f="") -> (s? t:f=w333:string)
        n105 = call <vilib>:"Add State(s) to Queue__JKI_lib_State_Machine.vi"("State(s) in (\"\")"=w333, "State(s) at Back (\"\")"="Data: Cleanup\nEvents: Unregister Events\nAction: Close Connection\nExit") -> ("States Out"=w331:string)  [unwired: 13 in]
        n106 = call <vilib>:"Add State(s) to Queue__JKI_lib_State_Machine.vi"("State(s) in Front (\"\")"=w331, "State(s) in (\"\")"=w340) -> ("States Out"=w339:string)  [unwired: 13 in]
      }
      frame "----------Action----------" {
        n107 = call <vilib>:"Add State(s) to Queue__JKI_lib_State_Machine.vi"("State(s) in (\"\")"=w345) -> ("States Out"=w344:string)  [unwired: 14 in]
      }
      frame "Action: Close Connection" {
        n108 = call <vilib>:"Add States to Queue using MultiLine String (no vData input).vi"("queue in"=w348, "states in"="Close TCP", "error in"=w346) -> ("error out"=w347:errorcluster)  [unwired: 10 in, 2 out]
        n109 = call <vilib>:"Add State(s) to Queue__JKI_lib_State_Machine.vi"("State(s) in (\"\")"=w353) -> ("States Out"=w352:string)  [unwired: 14 in]
      }
      frame "Process: Sync" {
        n110 = Unbundle By Name(w356) -> ("notifierSync"=w357:refnum<notifier>)
        n111 = Send Notification(notification=TRUE, notifier=w357, error in (no error)=w354) -> (error out=w355:errorcluster)  [unwired: 1 out]
        n112 = call <vilib>:"Add State(s) to Queue__JKI_lib_State_Machine.vi"("State(s) in (\"\")"=w361) -> ("States Out"=w360:string)  [unwired: 14 in]
      }
      frame "Action: CheckPollTimers" {
        n113 = Unbundle By Name(w371) -> ("PollTracker.HeadStatusPollStart"=w368:dbl)
        n114 = Unbundle By Name(w371) -> ("PollTimers.HeadStatus"=w366:dbl)
        n115 = Get Date/Time In Seconds() -> (seconds since 1Jan1904=w370:timestamp)
        n116 = To Double Precision Float(number=w370) -> (double precision float=w369:dbl)
        n117 = Subtract(x=w369, y=w368) -> (x-y=w367:dbl)
        n118 = Greater?(x=w367, y=w366) -> (0:w362:bool)
        n119 = Select(t="Action: Send GIS Command>>P,HT,R", s=w362, f="") -> (s? t:f=w363:string)
        n120 = call <vilib>:"Add State(s) to Queue__JKI_lib_State_Machine.vi"("State(s) in Front (\"\")"=w363, "State(s) in (\"\")"=w375) -> ("States Out"=w374:string)  [unwired: 13 in]
      }
      frame "Action: Start Poll" {
        n121 = Get Date/Time In Seconds() -> (seconds since 1Jan1904=w377:timestamp)
        n122 = To Double Precision Float(number=w377) -> (double precision float=w376:dbl)
        n123 = Bundle By Name(cluster=w381, "PollTracker.Poll"=TRUE, "PollTracker.HeadStatusPollStart"=w376) -> (w379:T7)
        n124 = call <vilib>:"Add State(s) to Queue__JKI_lib_State_Machine.vi"("State(s) in (\"\")"=w384) -> ("States Out"=w383:string)  [unwired: 14 in]
      }
      frame "Events: Register Events" {
        n125 = call-dynamic "GetEvents_TopLevel.vi"("error in (no error)"=w386, "TopLevel in"=w388) -> ("error out"=w387:errorcluster, "UserEvents"=w389:T19)  [unwired: 7 in, 1 out]
        n126 = Unbundle By Name(w394) -> ("GIS Printer in"=w395:refnum<class "GIS Printer.lvclass">)
        n127 = Unbundle By Name(w389) -> ("AppEvent"=w385:refnum<user-event>)
        n128 = call-dynamic "GetEvents_GIS Printer.vi"("error in (no error)"=w387, "TopLevel in"=w395) -> ("error out"=w390:errorcluster, "UserEvents"=w393:T20)  [unwired: 7 in, 1 out]
        n129 = Unbundle By Name(w393) -> ("Abort"=w392:refnum<user-event>, "stop process"=w391:refnum<user-event>)
        n130 = register-events(w397, w392, w391, w385) -> (reference out=w396:refnum<event-registration>)  [unwired: 2 in, 1 out]
        n131 = call <vilib>:"Add State(s) to Queue__JKI_lib_State_Machine.vi"("State(s) in (\"\")"=w399) -> ("States Out"=w398:string)  [unwired: 14 in]
      }
      frame "Events: Unregister Events" {
        n132 = Unregister For Events(event registration refnum=w402, error in=w400) -> (error out=w401:errorcluster)
        n133 = call <vilib>:"Add State(s) to Queue__JKI_lib_State_Machine.vi"("State(s) in (\"\")"=w405) -> ("States Out"=w404:string)  [unwired: 14 in]
      }
      frame "Action: Send GIS Command" {
        n134 = Get Date/Time In Seconds() -> (seconds since 1Jan1904=w407:timestamp)
        n135 = To Double Precision Float(number=w407) -> (double precision float=w406:dbl)
        n136 = call <vilib>:"Add State to Queue with vData.vi"("queue in"=w412, "state in"="SendCmdToPrinter", "vData (\"\")"=w413, "error in"=w410) -> ("error out"=w411:errorcluster)  [unwired: 8 in, 3 out]
        n137 = Bundle By Name(cluster=w415, "PollTracker.HeadStatusPollStart"=w406) -> (w408:T7)
        n138 = call <vilib>:"Add State(s) to Queue__JKI_lib_State_Machine.vi"("State(s) in (\"\")"=w417) -> ("States Out"=w416:string)  [unwired: 14 in]
      }
      frame "Action: Open Connection" {
        n139 = disable-structure shown="Enabled" {
          disable-tunnel: w420 -> [w435 w436]
          disable-tunnel: w418 -> [w434 _]
          disable-tunnel: [w432 w436] -> w425
          disable-tunnel: [w431 refnum<k5> refnum ("connection ID")] -> w424
          frame Enabled {
            (unwired) "localhost" ("address")
            n140 = Unbundle By Name(w434) -> ("PrinterConfiguration.IPAddress"=w429:string)
            n141 = TCP Open Connection(address=w429, remote port or service name=u16 2000, timeout ms (60000)=1000, error in (no error)=w435) -> (connection ID=w431:refnum<k5>, error out=w432:errorcluster)  [unwired: 1 in]
          }
          frame Disabled {
          }
        }
        n142 = call <vilib>:"Add State to Queue with vData.vi"("queue in"=w422, "state in"="UpdateSettings>>TCP", "vData (\"\")"=w424, "error in"=w425) -> ("error out"=w421:errorcluster)  [unwired: 8 in, 3 out]
        n143 = Bundle By Name(cluster=w418, "TCP"=w424) -> (w419:T7)
        n144 = call <vilib>:"Add State(s) to Queue__JKI_lib_State_Machine.vi"("State(s) in (\"\")"=w428) -> ("States Out"=w427:string)  [unwired: 14 in]
      }
    }
  }
  n145 = disable-structure shown="Enabled" {
    disable-tunnel: w18 -> [w441 w574 w880]
    disable-tunnel: w15 -> [w440 w573 w879]
    disable-tunnel: w14 -> [w439 w572 w878]
    disable-tunnel: [w438 _ _] -> w11
    frame Enabled {
      n146 = while {
        tunnel: w439 -> [w447]
        shift-right: [w451] -> w438
        shift-left: w441 -> [w453]
        shift-right: [w448] -> _
        shift-left: w440 -> [w449]
        stop <- w454 stop-if-true
        n147 = call <vilib>:"Get Next Queued State with vData.vi"("queue in"=w447, "error in (no error)"=w453) -> ("vData out"=w450:variant, "queue out"=w446:refnum<queue>, "Next State"=w445:string, "queued msg"=w442:string, "error out"=w452:errorcluster)  [unwired: 7 in, 2 out]
        n148 = call <vilib>:"Parse State Queue__JKI_lib_State_Machine.vi"("State Queue"=w445) -> ("Current State"=w444:string, "Arguments"=w443:string)  [unwired: 12 in, 1 out]
        n149 = case shown="\"\", \"EventHandler\", \"Idle\"" w444 {
          tunnel: [_ _ _ _ _ _ _ _ TRUE] -> w454
          tunnel: w452 -> [w456 w460 w476 w500 w504 w539 w545 w565 w570]
          tunnel: [w456 w457 w466 w500 w503 errorcluster {"status"=FALSE, "code"=0, "source"=""} ("error out") w544 w564 w570] -> w451
          tunnel: w450 -> [_ _ w474 _ _ _ w546 _ _]
          tunnel: w449 -> [w455 w462 w471 w499 w502 w538 w543 w568 w569]
          tunnel: [w455 w459 w469 w498 w501 w538 w542 w563 w569] -> w448
          tunnel: w446 -> [_ _ _ _ _ _ _ w567 _]
          tunnel: w443 -> [_ _ _ _ _ _ _ _ _]
          tunnel: w442 -> [_ _ _ _ _ _ w541 _ _]
          frame Default {
          }
          frame "Close TCP" {
            n150 = Unbundle By Name(w462) -> ("TCP"=w463:refnum<k5>)
            n151 = TCP Close Connection(connection ID=w463, error in (no error)=w460) -> (error out=w461:errorcluster)  [unwired: 1 in, 1 out]
            n152 = call <vilib>:"Clear Errors.vi"("error in (no error)"=w461) -> ("error out"=w457:errorcluster)  [unwired: 5 in, 1 out]
            n153 = Bundle By Name(cluster=w462, "Open"=FALSE) -> (w459:T1)
          }
          frame "SendCmdToPrinter" {
            n154 = Variant To Data(error in=w476, type="", Variant=w474) -> (data=w473:string, error out=w472:errorcluster)
            n155 = Unbundle By Name(w471) -> ("TCP"=w470:refnum<k5>)
            n156 = Concatenate Strings(w473, "\n") -> (w465:string)
            n157 = disable-structure shown="Enabled" {
              disable-tunnel: w470 -> [w494 w496]
              disable-tunnel: [w493 w496] -> w468
              disable-tunnel: w472 -> [w491 w495]
              disable-tunnel: w465 -> [w490 _]
              disable-tunnel: [w489 w495] -> w467
              disable-tunnel: [w488 _] -> _
              frame Enabled {
                n158 = TCP Write(connection ID=w494, data in=w490, error in (no error)=w491, 9:100 ("timeout ms (25000)")) -> (connection ID out=w493:refnum<k5>, bytes written=w488:i32, error out=w489:errorcluster)
              }
              frame Disabled {
              }
            }
            n159 = disable-structure shown="Disabled" {
              disable-tunnel: w471 -> [w485 w487]
              disable-tunnel: [w484 w487] -> w469
              disable-tunnel: w468 -> [w481 _]
              disable-tunnel: w467 -> [w480 w486]
              disable-tunnel: [w479 w486] -> w466
              frame Disabled {
                n160 = TCP Read(connection ID=w481, bytes to read=100, error in (no error)=w480, 9:1000 ("timeout ms (25000)")) -> (connection ID out=w477:refnum<k5>, data out=w478:string, error out=w479:errorcluster)  [unwired: 1 in]
                n161 = Bundle By Name(cluster=w485, "TCP"=w477) -> (w484:T1)
                n162 = flat-sequence {
                  tunnel: w478 -> [_]
                  frame #0 {
                  }
                }
              }
              frame Enabled {
              }
            }
          }
          frame "Initialize" {
            n163 = Bundle By Name(cluster=w499, "Open"=FALSE) -> (w498:T1)
          }
          frame "", "EventHandler", "Idle" {
            n164 = event shown="[0] Timeout" {
              selector: _ -> [_]
              dyn-events: _ -> [_]
              timeout: 1 -> [_]
              tunnel: w502 -> [w509]
              tunnel: w504 -> [w507]
              tunnel: [w506] -> w503
              tunnel: [w510] -> w501
              event Timeout {
                n165 = event-data() -> ()  [unwired: 1 in, 3 out]
                n166 = Unbundle By Name(w509) -> ("Open"=w508:bool)
                n167 = case shown="True" w508 {
                  tunnel: w509 -> [w512 w526]
                  tunnel: [w512 w524] -> w510
                  tunnel: w507 -> [w511 w514]
                  tunnel: [w511 w513] -> w506
                  frame False {
                  }
                  frame True {
                    n168 = Unbundle By Name(w526) -> ("String"=w525:string, "PrinterPollResponse"=w522:refnum<user-event>, "TCP"=w521:refnum<k5>)
                    n169 = TCP Read(connection ID=w521, bytes to read=500, error in (no error)=w514, 9:100 ("timeout ms (25000)")) -> (connection ID out=w515:refnum<k5>, data out=w520:string, error out=w516:errorcluster)  [unwired: 1 in]
                    n170 = Empty String/Path?(string/path=w520) -> (empty?=w519:bool)
                    n171 = case shown="True" w519 {
                      tunnel: w525 -> [w533 w536]
                      tunnel: [w532 w537] -> w523
                      tunnel: w522 -> [w531 w535]
                      tunnel: w520 -> [w530 _]
                      frame False {
                        n172 = Concatenate Strings(w533, w530) -> (w534:string)
                        n173 = call "ProcessSerialData.vi"("SerialResponseEvent"=w531, "String in"=w534) -> ("String out"=w532:string)  [unwired: 9 in]
                      }
                      frame True {
                        n174 = call "ProcessSerialData.vi"("SerialResponseEvent"=w535, "String in"=w536) -> ("String out"=w537:string)  [unwired: 9 in]
                      }
                    }
                    n175 = flat-sequence {
                      tunnel: w516 -> [w529]
                      tunnel: [w527] -> w513
                      frame #0 {
                        # "#todo handle error 56"
                        n176 = call <vilib>:"Clear Errors.vi"("error in (no error)"=w529, "specific error code to clear (0: all)"=56) -> ("error out"=w527:errorcluster)  [unwired: 4 in, 1 out]
                      }
                    }
                    n177 = Bundle By Name(cluster=w526, "String"=w523, "TCP"=w515) -> (w524:T1)
                  }
                }
              }
            }
          }
          frame "Error Handler" {
            n178 = call <vilib>:"General Error Handler.vi"("error in (no error)"=w539) -> ()  [unwired: 10 in, 5 out]
          }
          frame "UpdateSettings" {
            n179 = case shown="\"Configuration\"" w541 {
              tunnel: w546 -> [_ w550 w558]
              tunnel: w545 -> [w548 w551 w559]
              tunnel: [w548 w552 w560] -> w544
              tunnel: w543 -> [w547 w553 w561]
              tunnel: [w547 w553 w556] -> w542
              frame "False", Default {
              }
              frame "Configuration" {
                n180 = Variant To Data(error in=w551, type="placeholder", Variant=w550) -> (error out=w552:errorcluster)  [unwired: 1 out]
              }
              frame "TCP" {
                w557 = refnum<k5> refnum  # TCP
                n181 = Variant To Data(error in=w559, type=w557, Variant=w558) -> (data=w555:refnum<k5>, error out=w560:errorcluster)
                n182 = Bundle By Name(cluster=w561, "TCP"=w555, "Open"=TRUE) -> (w556:T1)
              }
            }
          }
          frame "Macro: Exit" {
            n183 = Bundle By Name(cluster=w568, "Open"=FALSE) -> (w563:T1)
            n184 = call <vilib>:"Add States to Queue using MultiLine String (no vData input).vi"("queue in"=w567, "states in"="Quit", "error in"=w565) -> ("error out"=w564:errorcluster)  [unwired: 10 in, 2 out]
          }
          frame "Quit" {
          }
        }
      }
    }
    frame Disabled {
      n185 = while {
        tunnel: w572 -> [w580]
        shift-right: [w584] -> _
        shift-left: w574 -> [w586]
        shift-right: [w581] -> _
        shift-left: w573 -> [w582]
        stop <- w587 stop-if-true
        n186 = call <vilib>:"Get Next Queued State with vData.vi"("queue in"=w580, "error in (no error)"=w586) -> ("vData out"=w583:variant, "queue out"=w579:refnum<queue>, "Next State"=w578:string, "queued msg"=w575:string, "error out"=w585:errorcluster)  [unwired: 7 in, 2 out]
        n187 = call <vilib>:"Parse State Queue__JKI_lib_State_Machine.vi"("State Queue"=w578) -> ("Current State"=w577:string, "Arguments"=w576:string)  [unwired: 12 in, 1 out]
        n188 = case shown="\"\", \"EventHandler\", \"Idle\"" w577 {
          tunnel: [_ _ _ _ _ _ _ TRUE] -> w587
          tunnel: w585 -> [w589 w602 w626 w630 w847 w853 w871 w876]
          tunnel: [w589 w592 w626 w629 errorcluster {"status"=FALSE, "code"=0, "source"=""} ("error out") w852 w870 w876] -> w584
          tunnel: w583 -> [_ w600 _ _ _ w854 _ _]
          tunnel: w582 -> [w588 w597 w625 w628 w846 w851 w874 w875]
          tunnel: [w588 w595 w624 w627 w846 w850 w874 w875] -> w581
          tunnel: w579 -> [_ _ _ _ _ _ w873 _]
          tunnel: w576 -> [_ _ _ _ _ _ _ _]
          tunnel: w575 -> [_ _ _ _ _ w849 _ _]
          frame Default {
          }
          frame "SendCmdToPrinter" {
            n189 = Variant To Data(error in=w602, type="", Variant=w600) -> (data=w599:string, error out=w598:errorcluster)
            n190 = Unbundle By Name(w597) -> ("TCP"=w596:refnum<k5>)
            n191 = Concatenate Strings(w599, "\n") -> (w591:string)
            n192 = disable-structure shown="Enabled" {
              disable-tunnel: w596 -> [w620 w622]
              disable-tunnel: [w619 w622] -> w594
              disable-tunnel: w598 -> [w617 w621]
              disable-tunnel: w591 -> [w616 _]
              disable-tunnel: [w615 w621] -> w593
              disable-tunnel: [w614 _] -> _
              frame Disabled {
                n193 = TCP Write(connection ID=w620, data in=w616, error in (no error)=w617, 9:100 ("timeout ms (25000)")) -> (connection ID out=w619:refnum<k5>, bytes written=w614:i32, error out=w615:errorcluster)
              }
              frame Enabled {
              }
            }
            n194 = disable-structure shown="Enabled" {
              disable-tunnel: w597 -> [w611 w613]
              disable-tunnel: [w610 w613] -> w595
              disable-tunnel: w594 -> [w607 _]
              disable-tunnel: w593 -> [w606 w612]
              disable-tunnel: [w605 w612] -> w592
              frame Disabled {
                n195 = TCP Read(connection ID=w607, bytes to read=100, error in (no error)=w606, 9:1000 ("timeout ms (25000)")) -> (connection ID out=w603:refnum<k5>, data out=w604:string, error out=w605:errorcluster)  [unwired: 1 in]
                n196 = Bundle By Name(cluster=w611, "TCP"=w603) -> (w610:T1)
                n197 = flat-sequence {
                  tunnel: w604 -> [_]
                  frame #0 {
                  }
                }
              }
              frame Enabled {
              }
            }
          }
          frame "Initialize" {
            n198 = Bundle By Name(cluster=w625, "Open"=FALSE) -> (w624:T1)
          }
          frame "", "EventHandler", "Idle" {
            n199 = event shown="[0] Timeout" {
              selector: _ -> [_ _ _ _ _ _ _ _ _ _]
              dyn-events: _ -> [_ _ _ _ _ _ _ _ _ _]
              timeout: 1 -> [_ _ _ _ _ _ _ _ _ _]
              tunnel: w628 -> [w633 w658 w679 w700 w721 w742 w763 w784 w805 w826]
              tunnel: w630 -> [w635 w660 w681 w702 w723 w744 w765 w786 w807 w828]
              tunnel: [w635 w660 w681 w702 w723 w744 w765 w786 w807 w828] -> w629
              tunnel: [w634 w659 w680 w701 w722 w743 w764 w785 w806 w827] -> w627
              event Timeout {
                n200 = event-data() -> ()  [unwired: 1 in, 3 out]
                n201 = Unbundle By Name(w633) -> ("Open"=w632:bool)
                n202 = case shown="True" w632 {
                  tunnel: w633 -> [w636 w648]
                  tunnel: [w636 w646] -> w634
                  frame False {
                  }
                  frame True {
                    n203 = Unbundle By Name(w648) -> ("String"=w647:string, "PrinterPollResponse"=w644:refnum<user-event>, "TCP"=w643:refnum<k5>)
                    n204 = TCP Read(connection ID=w643, bytes to read=500, 9:100 ("timeout ms (25000)")) -> (connection ID out=w637:refnum<k5>, data out=w642:string, error out=w638:errorcluster)  [unwired: 2 in]
                    n205 = Empty String/Path?(string/path=w642) -> (empty?=w641:bool)
                    n206 = case shown="False" w641 {
                      tunnel: w647 -> [w652 w655]
                      tunnel: [w651 w656] -> w645
                      tunnel: w644 -> [w650 w654]
                      tunnel: w642 -> [w649 _]
                      frame False {
                        n207 = Concatenate Strings(w652, w649) -> (w653:string)
                        n208 = call "ProcessSerialData.vi"("SerialResponseEvent"=w650, "String in"=w653) -> ("String out"=w651:string)  [unwired: 9 in]
                      }
                      frame True {
                        n209 = call "ProcessSerialData.vi"("SerialResponseEvent"=w654, "String in"=w655) -> ("String out"=w656:string)  [unwired: 9 in]
                      }
                    }
                    n210 = flat-sequence {
                      tunnel: w638 -> [_]
                      frame #0 {
                        # "#todo handle error 56"
                      }
                    }
                    n211 = Bundle By Name(cluster=w648, "String"=w645, "TCP"=w637) -> (w646:T1)
                  }
                }
              }
              event "A11": Value Change {
                n212 = event-data() -> ()  [unwired: 1 in, 6 out]
                n213 = Unbundle By Name(w658) -> ("Open"=w657:bool)
                n214 = case shown="True" w657 {
                  tunnel: w658 -> [w661 w669]
                  tunnel: [w661 w667] -> w659
                  frame False {
                  }
                  frame True {
                    w662 = "A,11,P,C,P,\"Print Manager,Print Line Manager,PMB-KM,PrintGoSource\",\"TTL\"\n"
                    n215 = Unbundle By Name(w669) -> ("String"=w668:string, "PrinterPollResponse"=w665:refnum<user-event>, "TCP"=w663:refnum<k5>)
                    n216 = Empty String/Path?(string/path=w662) -> (empty?=w664:bool)
                    n217 = case shown="False" w664 {
                      tunnel: w668 -> [w673 w676]
                      tunnel: [w672 w677] -> w666
                      tunnel: w665 -> [w671 w675]
                      tunnel: w662 -> [w670 _]
                      frame False {
                        n218 = Concatenate Strings(w673, w670) -> (w674:string)
                        n219 = call "ProcessSerialData.vi"("SerialResponseEvent"=w671, "String in"=w674) -> ("String out"=w672:string)  [unwired: 9 in]
                      }
                      frame True {
                        n220 = call "ProcessSerialData.vi"("SerialResponseEvent"=w675, "String in"=w676) -> ("String out"=w677:string)  [unwired: 9 in]
                      }
                    }
                    n221 = Bundle By Name(cluster=w669, "String"=w666, "TCP"=w663) -> (w667:T1)
                  }
                }
              }
              event "C11": Value Change {
                n222 = event-data() -> ()  [unwired: 1 in, 6 out]
                n223 = Unbundle By Name(w679) -> ("Open"=w678:bool)
                n224 = case shown="True" w678 {
                  tunnel: w679 -> [w682 w690]
                  tunnel: [w682 w688] -> w680
                  frame False {
                  }
                  frame True {
                    w683 = "C,11,0\n"
                    n225 = Unbundle By Name(w690) -> ("String"=w689:string, "PrinterPollResponse"=w686:refnum<user-event>, "TCP"=w684:refnum<k5>)
                    n226 = Empty String/Path?(string/path=w683) -> (empty?=w685:bool)
                    n227 = case shown="True" w685 {
                      tunnel: w689 -> [w694 w697]
                      tunnel: [w693 w698] -> w687
                      tunnel: w686 -> [w692 w696]
                      tunnel: w683 -> [w691 _]
                      frame False {
                        n228 = Concatenate Strings(w694, w691) -> (w695:string)
                        n229 = call "ProcessSerialData.vi"("SerialResponseEvent"=w692, "String in"=w695) -> ("String out"=w693:string)  [unwired: 9 in]
                      }
                      frame True {
                        n230 = call "ProcessSerialData.vi"("SerialResponseEvent"=w696, "String in"=w697) -> ("String out"=w698:string)  [unwired: 9 in]
                      }
                    }
                    n231 = Bundle By Name(cluster=w690, "String"=w687, "TCP"=w684) -> (w688:T1)
                  }
                }
              }
              event "A22": Value Change {
                n232 = event-data() -> ()  [unwired: 1 in, 6 out]
                n233 = Unbundle By Name(w700) -> ("Open"=w699:bool)
                n234 = case shown="True" w699 {
                  tunnel: w700 -> [w703 w711]
                  tunnel: [w703 w709] -> w701
                  frame False {
                  }
                  frame True {
                    w704 = "A,22,P,C,P,\"Print Manager,Print Line Manager,PMB-KM,EncoderSource\",\"RS422\"\n"
                    n235 = Unbundle By Name(w711) -> ("String"=w710:string, "PrinterPollResponse"=w707:refnum<user-event>, "TCP"=w705:refnum<k5>)
                    n236 = Empty String/Path?(string/path=w704) -> (empty?=w706:bool)
                    n237 = case shown="True" w706 {
                      tunnel: w710 -> [w715 w718]
                      tunnel: [w714 w719] -> w708
                      tunnel: w707 -> [w713 w717]
                      tunnel: w704 -> [w712 _]
                      frame False {
                        n238 = Concatenate Strings(w715, w712) -> (w716:string)
                        n239 = call "ProcessSerialData.vi"("SerialResponseEvent"=w713, "String in"=w716) -> ("String out"=w714:string)  [unwired: 9 in]
                      }
                      frame True {
                        n240 = call "ProcessSerialData.vi"("SerialResponseEvent"=w717, "String in"=w718) -> ("String out"=w719:string)  [unwired: 9 in]
                      }
                    }
                    n241 = Bundle By Name(cluster=w711, "String"=w708, "TCP"=w705) -> (w709:T1)
                  }
                }
              }
              event "C22": Value Change {
                n242 = event-data() -> ()  [unwired: 1 in, 6 out]
                n243 = Unbundle By Name(w721) -> ("Open"=w720:bool)
                n244 = case shown="True" w720 {
                  tunnel: w721 -> [w724 w732]
                  tunnel: [w724 w730] -> w722
                  frame False {
                  }
                  frame True {
                    w725 = "C,22,0\n"
                    n245 = Unbundle By Name(w732) -> ("String"=w731:string, "PrinterPollResponse"=w728:refnum<user-event>, "TCP"=w726:refnum<k5>)
                    n246 = Empty String/Path?(string/path=w725) -> (empty?=w727:bool)
                    n247 = case shown="True" w727 {
                      tunnel: w731 -> [w736 w739]
                      tunnel: [w735 w740] -> w729
                      tunnel: w728 -> [w734 w738]
                      tunnel: w725 -> [w733 _]
                      frame False {
                        n248 = Concatenate Strings(w736, w733) -> (w737:string)
                        n249 = call "ProcessSerialData.vi"("SerialResponseEvent"=w734, "String in"=w737) -> ("String out"=w735:string)  [unwired: 9 in]
                      }
                      frame True {
                        n250 = call "ProcessSerialData.vi"("SerialResponseEvent"=w738, "String in"=w739) -> ("String out"=w740:string)  [unwired: 9 in]
                      }
                    }
                    n251 = Bundle By Name(cluster=w732, "String"=w729, "TCP"=w726) -> (w730:T1)
                  }
                }
              }
              event "A33": Value Change {
                n252 = event-data() -> ()  [unwired: 1 in, 6 out]
                n253 = Unbundle By Name(w742) -> ("Open"=w741:bool)
                n254 = case shown="True" w741 {
                  tunnel: w742 -> [w745 w753]
                  tunnel: [w745 w751] -> w743
                  frame False {
                  }
                  frame True {
                    w746 = "A,33,P,P,1,C:\\Users\\labuser\\Desktop\\Scripts\\Patterns\\Print Weights\\PH1\\PW.bmp,5\n"
                    n255 = Unbundle By Name(w753) -> ("String"=w752:string, "PrinterPollResponse"=w749:refnum<user-event>, "TCP"=w747:refnum<k5>)
                    n256 = Empty String/Path?(string/path=w746) -> (empty?=w748:bool)
                    n257 = case shown="True" w748 {
                      tunnel: w752 -> [w757 w760]
                      tunnel: [w756 w761] -> w750
                      tunnel: w749 -> [w755 w759]
                      tunnel: w746 -> [w754 _]
                      frame False {
                        n258 = Concatenate Strings(w757, w754) -> (w758:string)
                        n259 = call "ProcessSerialData.vi"("SerialResponseEvent"=w755, "String in"=w758) -> ("String out"=w756:string)  [unwired: 9 in]
                      }
                      frame True {
                        n260 = call "ProcessSerialData.vi"("SerialResponseEvent"=w759, "String in"=w760) -> ("String out"=w761:string)  [unwired: 9 in]
                      }
                    }
                    n261 = Bundle By Name(cluster=w753, "String"=w750, "TCP"=w747) -> (w751:T1)
                  }
                }
              }
              event "I33 1": Value Change {
                n262 = event-data() -> ()  [unwired: 1 in, 6 out]
                n263 = Unbundle By Name(w763) -> ("Open"=w762:bool)
                n264 = case shown="True" w762 {
                  tunnel: w763 -> [w766 w774]
                  tunnel: [w766 w772] -> w764
                  frame False {
                  }
                  frame True {
                    w767 = "I,33,P\n"
                    n265 = Unbundle By Name(w774) -> ("String"=w773:string, "PrinterPollResponse"=w770:refnum<user-event>, "TCP"=w768:refnum<k5>)
                    n266 = Empty String/Path?(string/path=w767) -> (empty?=w769:bool)
                    n267 = case shown="True" w769 {
                      tunnel: w773 -> [w778 w781]
                      tunnel: [w777 w782] -> w771
                      tunnel: w770 -> [w776 w780]
                      tunnel: w767 -> [w775 _]
                      frame False {
                        n268 = Concatenate Strings(w778, w775) -> (w779:string)
                        n269 = call "ProcessSerialData.vi"("SerialResponseEvent"=w776, "String in"=w779) -> ("String out"=w777:string)  [unwired: 9 in]
                      }
                      frame True {
                        n270 = call "ProcessSerialData.vi"("SerialResponseEvent"=w780, "String in"=w781) -> ("String out"=w782:string)  [unwired: 9 in]
                      }
                    }
                    n271 = Bundle By Name(cluster=w774, "String"=w771, "TCP"=w768) -> (w772:T1)
                  }
                }
              }
              event "I33 2": Value Change {
                n272 = event-data() -> ()  [unwired: 1 in, 6 out]
                n273 = Unbundle By Name(w784) -> ("Open"=w783:bool)
                n274 = case shown="True" w783 {
                  tunnel: w784 -> [w787 w795]
                  tunnel: [w787 w793] -> w785
                  frame False {
                  }
                  frame True {
                    w788 = "I,33,RTP,1\n"
                    n275 = Unbundle By Name(w795) -> ("String"=w794:string, "PrinterPollResponse"=w791:refnum<user-event>, "TCP"=w789:refnum<k5>)
                    n276 = Empty String/Path?(string/path=w788) -> (empty?=w790:bool)
                    n277 = case shown="True" w790 {
                      tunnel: w794 -> [w799 w802]
                      tunnel: [w798 w803] -> w792
                      tunnel: w791 -> [w797 w801]
                      tunnel: w788 -> [w796 _]
                      frame False {
                        n278 = Concatenate Strings(w799, w796) -> (w800:string)
                        n279 = call "ProcessSerialData.vi"("SerialResponseEvent"=w797, "String in"=w800) -> ("String out"=w798:string)  [unwired: 9 in]
                      }
                      frame True {
                        n280 = call "ProcessSerialData.vi"("SerialResponseEvent"=w801, "String in"=w802) -> ("String out"=w803:string)  [unwired: 9 in]
                      }
                    }
                    n281 = Bundle By Name(cluster=w795, "String"=w792, "TCP"=w789) -> (w793:T1)
                  }
                }
              }
              event "I33 3": Value Change {
                n282 = event-data() -> ()  [unwired: 1 in, 6 out]
                n283 = Unbundle By Name(w805) -> ("Open"=w804:bool)
                n284 = case shown="True" w804 {
                  tunnel: w805 -> [w808 w816]
                  tunnel: [w808 w814] -> w806
                  frame False {
                  }
                  frame True {
                    w809 = "I,33,EP\n"
                    n285 = Unbundle By Name(w816) -> ("String"=w815:string, "PrinterPollResponse"=w812:refnum<user-event>, "TCP"=w810:refnum<k5>)
                    n286 = Empty String/Path?(string/path=w809) -> (empty?=w811:bool)
                    n287 = case shown="True" w811 {
                      tunnel: w815 -> [w820 w823]
                      tunnel: [w819 w824] -> w813
                      tunnel: w812 -> [w818 w822]
                      tunnel: w809 -> [w817 _]
                      frame False {
                        n288 = Concatenate Strings(w820, w817) -> (w821:string)
                        n289 = call "ProcessSerialData.vi"("SerialResponseEvent"=w818, "String in"=w821) -> ("String out"=w819:string)  [unwired: 9 in]
                      }
                      frame True {
                        n290 = call "ProcessSerialData.vi"("SerialResponseEvent"=w822, "String in"=w823) -> ("String out"=w824:string)  [unwired: 9 in]
                      }
                    }
                    n291 = Bundle By Name(cluster=w816, "String"=w813, "TCP"=w810) -> (w814:T1)
                  }
                }
              }
              event "C33": Value Change {
                n292 = event-data() -> ()  [unwired: 1 in, 6 out]
                n293 = Unbundle By Name(w826) -> ("Open"=w825:bool)
                n294 = case shown="True" w825 {
                  tunnel: w826 -> [w829 w837]
                  tunnel: [w829 w835] -> w827
                  frame False {
                  }
                  frame True {
                    w830 = "C,33,0\n"
                    n295 = Unbundle By Name(w837) -> ("String"=w836:string, "PrinterPollResponse"=w833:refnum<user-event>, "TCP"=w831:refnum<k5>)
                    n296 = Empty String/Path?(string/path=w830) -> (empty?=w832:bool)
                    n297 = case shown="True" w832 {
                      tunnel: w836 -> [w841 w844]
                      tunnel: [w840 w845] -> w834
                      tunnel: w833 -> [w839 w843]
                      tunnel: w830 -> [w838 _]
                      frame False {
                        n298 = Concatenate Strings(w841, w838) -> (w842:string)
                        n299 = call "ProcessSerialData.vi"("SerialResponseEvent"=w839, "String in"=w842) -> ("String out"=w840:string)  [unwired: 9 in]
                      }
                      frame True {
                        n300 = call "ProcessSerialData.vi"("SerialResponseEvent"=w843, "String in"=w844) -> ("String out"=w845:string)  [unwired: 9 in]
                      }
                    }
                    n301 = Bundle By Name(cluster=w837, "String"=w834, "TCP"=w831) -> (w835:T1)
                  }
                }
              }
            }
          }
          frame "Error Handler" {
            n302 = call <vilib>:"General Error Handler.vi"("error in (no error)"=w847) -> ()  [unwired: 10 in, 5 out]
          }
          frame "UpdateSettings" {
            n303 = case shown="\"TCP\"" w849 {
              tunnel: w854 -> [_ w858 w866]
              tunnel: w853 -> [w856 w859 w867]
              tunnel: [w856 w860 w868] -> w852
              tunnel: w851 -> [w855 w861 w869]
              tunnel: [w855 w861 w864] -> w850
              frame "False", Default {
              }
              frame "Configuration" {
                n304 = Variant To Data(error in=w859, type="placeholder", Variant=w858) -> (error out=w860:errorcluster)  [unwired: 1 out]
              }
              frame "TCP" {
                w865 = refnum<k5> refnum  # TCP
                n305 = Variant To Data(error in=w867, type=w865, Variant=w866) -> (data=w863:refnum<k5>, error out=w868:errorcluster)
                n306 = Bundle By Name(cluster=w869, "TCP"=w863, "Open"=TRUE) -> (w864:T1)
              }
            }
          }
          frame "Macro: Exit" {
            n307 = call <vilib>:"Add States to Queue using MultiLine String (no vData input).vi"("queue in"=w873, "states in"="Quit", "error in"=w871) -> ("error out"=w870:errorcluster)  [unwired: 10 in, 2 out]
          }
          frame "Quit" {
          }
        }
      }
    }
    frame Disabled {
      n308 = while {
        tunnel: w878 -> [w886]
        shift-right: [w890] -> _
        shift-left: w880 -> [w892]
        shift-right: [w887] -> _
        shift-left: w879 -> [w888]
        stop <- w893 stop-if-true
        n309 = call <vilib>:"Get Next Queued State with vData.vi"("queue in"=w886, "error in (no error)"=w892) -> ("vData out"=w889:variant, "queue out"=w885:refnum<queue>, "Next State"=w884:string, "queued msg"=w881:string, "error out"=w891:errorcluster)  [unwired: 7 in, 2 out]
        n310 = call <vilib>:"Parse State Queue__JKI_lib_State_Machine.vi"("State Queue"=w884) -> ("Current State"=w883:string, "Arguments"=w882:string)  [unwired: 12 in, 1 out]
        n311 = case shown="\"\", \"EventHandler\", \"Idle\"" w883 {
          tunnel: [_ _ _ _ _ _ TRUE] -> w893
          tunnel: w891 -> [w895 w899 w903 w1069 w1075 w1093 w1098]
          tunnel: [w895 w899 w902 errorcluster {"status"=FALSE, "code"=0, "source"=""} ("error out") w1074 w1092 w1098] -> w890
          tunnel: w889 -> [_ _ _ _ w1076 _ _]
          tunnel: w888 -> [w894 w898 w901 w1068 w1073 w1096 w1097]
          tunnel: [w894 w897 w900 w1068 w1072 w1096 w1097] -> w887
          tunnel: w885 -> [_ _ _ _ _ w1095 _]
          tunnel: w882 -> [_ _ _ _ _ _ _]
          tunnel: w881 -> [_ _ _ _ w1071 _ _]
          frame Default {
          }
          frame "Initialize" {
            n312 = Bundle By Name(cluster=w898, "Open"=FALSE) -> (w897:T1)
          }
          frame "", "EventHandler", "Idle" {
            n313 = event shown="[1] \"A4\": Value Change" {
              selector: _ -> [_ _ _ _ _ _ _ _ _]
              dyn-events: _ -> [_ _ _ _ _ _ _ _ _]
              timeout: 1 -> [_ _ _ _ _ _ _ _ _]
              tunnel: w901 -> [w906 w925 w943 w961 w979 w997 w1015 w1033 w1051]
              tunnel: w903 -> [w908 w927 w945 w963 w981 w999 w1017 w1035 w1053]
              tunnel: [w908 w927 w945 w963 w981 w999 w1017 w1035 w1053] -> w902
              tunnel: [w907 w926 w944 w962 w980 w998 w1016 w1034 w1052] -> w900
              event Timeout {
                n314 = event-data() -> ()  [unwired: 1 in, 3 out]
                n315 = Unbundle By Name(w906) -> ("Open"=w905:bool)
                n316 = case shown="True" w905 {
                  tunnel: w906 -> [w909 w917]
                  tunnel: [w909 w915] -> w907
                  frame False {
                  }
                  frame True {
                    n317 = Unbundle By Name(w917) -> ("String"=w916:string, "PrinterPollResponse"=w913:refnum<user-event>, "TCP"=w912:refnum<k5>)
                    n318 = TCP Read(connection ID=w912) -> (data out=w911:string)  [unwired: 4 in, 2 out]
                    n319 = Empty String/Path?(string/path=w911) -> (empty?=w910:bool)
                    n320 = case shown="True" w910 {
                      tunnel: w916 -> [w921 w923]
                      tunnel: [w920 w923] -> w914
                      tunnel: w913 -> [w919 _]
                      tunnel: w911 -> [w918 _]
                      frame False {
                        n321 = Concatenate Strings(w921, w918) -> (w922:string)
                        n322 = call "ProcessSerialData.vi"("SerialResponseEvent"=w919, "String in"=w922) -> ("String out"=w920:string)  [unwired: 9 in]
                      }
                      frame True {
                      }
                    }
                    n323 = Bundle By Name(cluster=w917, "String"=w914) -> (w915:T1)
                  }
                }
              }
              event "A4": Value Change {
                n324 = event-data() -> ()  [unwired: 1 in, 6 out]
                n325 = Unbundle By Name(w925) -> ("Open"=w924:bool)
                n326 = case shown="True" w924 {
                  tunnel: w925 -> [w928 w935]
                  tunnel: [w928 w933] -> w926
                  frame False {
                  }
                  frame True {
                    w929 = "A,44,P,V,P,PH4_Temp_Read\n"
                    n327 = Unbundle By Name(w935) -> ("String"=w934:string, "PrinterPollResponse"=w931:refnum<user-event>)
                    n328 = Empty String/Path?(string/path=w929) -> (empty?=w930:bool)
                    n329 = case shown="False" w930 {
                      tunnel: w934 -> [w939 w941]
                      tunnel: [w938 w941] -> w932
                      tunnel: w931 -> [w937 _]
                      tunnel: w929 -> [w936 _]
                      frame False {
                        n330 = Concatenate Strings(w939, w936) -> (w940:string)
                        n331 = call "ProcessSerialData.vi"("SerialResponseEvent"=w937, "String in"=w940) -> ("String out"=w938:string)  [unwired: 9 in]
                      }
                      frame True {
                      }
                    }
                    n332 = Bundle By Name(cluster=w935, "String"=w932) -> (w933:T1)
                  }
                }
              }
              event "C4": Value Change {
                n333 = event-data() -> ()  [unwired: 1 in, 6 out]
                n334 = Unbundle By Name(w943) -> ("Open"=w942:bool)
                n335 = case shown="True" w942 {
                  tunnel: w943 -> [w946 w953]
                  tunnel: [w946 w951] -> w944
                  frame False {
                  }
                  frame True {
                    w947 = "C,44,0,40\n"
                    n336 = Unbundle By Name(w953) -> ("String"=w952:string, "PrinterPollResponse"=w949:refnum<user-event>)
                    n337 = Empty String/Path?(string/path=w947) -> (empty?=w948:bool)
                    n338 = case shown="False" w948 {
                      tunnel: w952 -> [w957 w959]
                      tunnel: [w956 w959] -> w950
                      tunnel: w949 -> [w955 _]
                      tunnel: w947 -> [w954 _]
                      frame False {
                        n339 = Concatenate Strings(w957, w954) -> (w958:string)
                        n340 = call "ProcessSerialData.vi"("SerialResponseEvent"=w955, "String in"=w958) -> ("String out"=w956:string)  [unwired: 9 in]
                      }
                      frame True {
                      }
                    }
                    n341 = Bundle By Name(cluster=w953, "String"=w950) -> (w951:T1)
                  }
                }
              }
              event "A3": Value Change {
                n342 = event-data() -> ()  [unwired: 1 in, 6 out]
                n343 = Unbundle By Name(w961) -> ("Open"=w960:bool)
                n344 = case shown="True" w960 {
                  tunnel: w961 -> [w964 w971]
                  tunnel: [w964 w969] -> w962
                  frame False {
                  }
                  frame True {
                    w965 = "A,33,P,V,P,PH3_Temp_Read\n"
                    n345 = Unbundle By Name(w971) -> ("String"=w970:string, "PrinterPollResponse"=w967:refnum<user-event>)
                    n346 = Empty String/Path?(string/path=w965) -> (empty?=w966:bool)
                    n347 = case shown="False" w966 {
                      tunnel: w970 -> [w975 w977]
                      tunnel: [w974 w977] -> w968
                      tunnel: w967 -> [w973 _]
                      tunnel: w965 -> [w972 _]
                      frame False {
                        n348 = Concatenate Strings(w975, w972) -> (w976:string)
                        n349 = call "ProcessSerialData.vi"("SerialResponseEvent"=w973, "String in"=w976) -> ("String out"=w974:string)  [unwired: 9 in]
                      }
                      frame True {
                      }
                    }
                    n350 = Bundle By Name(cluster=w971, "String"=w968) -> (w969:T1)
                  }
                }
              }
              event "C3": Value Change {
                n351 = event-data() -> ()  [unwired: 1 in, 6 out]
                n352 = Unbundle By Name(w979) -> ("Open"=w978:bool)
                n353 = case shown="True" w978 {
                  tunnel: w979 -> [w982 w989]
                  tunnel: [w982 w987] -> w980
                  frame False {
                  }
                  frame True {
                    w983 = "C,33,0,30\n"
                    n354 = Unbundle By Name(w989) -> ("String"=w988:string, "PrinterPollResponse"=w985:refnum<user-event>)
                    n355 = Empty String/Path?(string/path=w983) -> (empty?=w984:bool)
                    n356 = case shown="False" w984 {
                      tunnel: w988 -> [w993 w995]
                      tunnel: [w992 w995] -> w986
                      tunnel: w985 -> [w991 _]
                      tunnel: w983 -> [w990 _]
                      frame False {
                        n357 = Concatenate Strings(w993, w990) -> (w994:string)
                        n358 = call "ProcessSerialData.vi"("SerialResponseEvent"=w991, "String in"=w994) -> ("String out"=w992:string)  [unwired: 9 in]
                      }
                      frame True {
                      }
                    }
                    n359 = Bundle By Name(cluster=w989, "String"=w986) -> (w987:T1)
                  }
                }
              }
              event "A2": Value Change {
                n360 = event-data() -> ()  [unwired: 1 in, 6 out]
                n361 = Unbundle By Name(w997) -> ("Open"=w996:bool)
                n362 = case shown="True" w996 {
                  tunnel: w997 -> [w1000 w1007]
                  tunnel: [w1000 w1005] -> w998
                  frame False {
                  }
                  frame True {
                    w1001 = "A,22,P,V,P,PH2_Temp_Read\n"
                    n363 = Unbundle By Name(w1007) -> ("String"=w1006:string, "PrinterPollResponse"=w1003:refnum<user-event>)
                    n364 = Empty String/Path?(string/path=w1001) -> (empty?=w1002:bool)
                    n365 = case shown="False" w1002 {
                      tunnel: w1006 -> [w1011 w1013]
                      tunnel: [w1010 w1013] -> w1004
                      tunnel: w1003 -> [w1009 _]
                      tunnel: w1001 -> [w1008 _]
                      frame False {
                        n366 = Concatenate Strings(w1011, w1008) -> (w1012:string)
                        n367 = call "ProcessSerialData.vi"("SerialResponseEvent"=w1009, "String in"=w1012) -> ("String out"=w1010:string)  [unwired: 9 in]
                      }
                      frame True {
                      }
                    }
                    n368 = Bundle By Name(cluster=w1007, "String"=w1004) -> (w1005:T1)
                  }
                }
              }
              event "C2": Value Change {
                n369 = event-data() -> ()  [unwired: 1 in, 6 out]
                n370 = Unbundle By Name(w1015) -> ("Open"=w1014:bool)
                n371 = case shown="True" w1014 {
                  tunnel: w1015 -> [w1018 w1025]
                  tunnel: [w1018 w1023] -> w1016
                  frame False {
                  }
                  frame True {
                    w1019 = "C,22,0,20\n"
                    n372 = Unbundle By Name(w1025) -> ("String"=w1024:string, "PrinterPollResponse"=w1021:refnum<user-event>)
                    n373 = Empty String/Path?(string/path=w1019) -> (empty?=w1020:bool)
                    n374 = case shown="False" w1020 {
                      tunnel: w1024 -> [w1029 w1031]
                      tunnel: [w1028 w1031] -> w1022
                      tunnel: w1021 -> [w1027 _]
                      tunnel: w1019 -> [w1026 _]
                      frame False {
                        n375 = Concatenate Strings(w1029, w1026) -> (w1030:string)
                        n376 = call "ProcessSerialData.vi"("SerialResponseEvent"=w1027, "String in"=w1030) -> ("String out"=w1028:string)  [unwired: 9 in]
                      }
                      frame True {
                      }
                    }
                    n377 = Bundle By Name(cluster=w1025, "String"=w1022) -> (w1023:T1)
                  }
                }
              }
              event "A1": Value Change {
                n378 = event-data() -> ()  [unwired: 1 in, 6 out]
                n379 = Unbundle By Name(w1033) -> ("Open"=w1032:bool)
                n380 = case shown="True" w1032 {
                  tunnel: w1033 -> [w1036 w1043]
                  tunnel: [w1036 w1041] -> w1034
                  frame False {
                  }
                  frame True {
                    w1037 = "A,11,P,V,P,PH1_Temp_Read\n"
                    n381 = Unbundle By Name(w1043) -> ("String"=w1042:string, "PrinterPollResponse"=w1039:refnum<user-event>)
                    n382 = Empty String/Path?(string/path=w1037) -> (empty?=w1038:bool)
                    n383 = case shown="False" w1038 {
                      tunnel: w1042 -> [w1047 w1049]
                      tunnel: [w1046 w1049] -> w1040
                      tunnel: w1039 -> [w1045 _]
                      tunnel: w1037 -> [w1044 _]
                      frame False {
                        n384 = Concatenate Strings(w1047, w1044) -> (w1048:string)
                        n385 = call "ProcessSerialData.vi"("SerialResponseEvent"=w1045, "String in"=w1048) -> ("String out"=w1046:string)  [unwired: 9 in]
                      }
                      frame True {
                      }
                    }
                    n386 = Bundle By Name(cluster=w1043, "String"=w1040) -> (w1041:T1)
                  }
                }
              }
              event "C1": Value Change {
                n387 = event-data() -> ()  [unwired: 1 in, 6 out]
                n388 = Unbundle By Name(w1051) -> ("Open"=w1050:bool)
                n389 = case shown="True" w1050 {
                  tunnel: w1051 -> [w1054 w1061]
                  tunnel: [w1054 w1059] -> w1052
                  frame False {
                  }
                  frame True {
                    w1055 = "C,11,0,10\n"
                    n390 = Unbundle By Name(w1061) -> ("String"=w1060:string, "PrinterPollResponse"=w1057:refnum<user-event>)
                    n391 = Empty String/Path?(string/path=w1055) -> (empty?=w1056:bool)
                    n392 = case shown="False" w1056 {
                      tunnel: w1060 -> [w1065 w1067]
                      tunnel: [w1064 w1067] -> w1058
                      tunnel: w1057 -> [w1063 _]
                      tunnel: w1055 -> [w1062 _]
                      frame False {
                        n393 = Concatenate Strings(w1065, w1062) -> (w1066:string)
                        n394 = call "ProcessSerialData.vi"("SerialResponseEvent"=w1063, "String in"=w1066) -> ("String out"=w1064:string)  [unwired: 9 in]
                      }
                      frame True {
                      }
                    }
                    n395 = Bundle By Name(cluster=w1061, "String"=w1058) -> (w1059:T1)
                  }
                }
              }
            }
          }
          frame "Error Handler" {
            n396 = call <vilib>:"General Error Handler.vi"("error in (no error)"=w1069) -> ()  [unwired: 10 in, 5 out]
          }
          frame "UpdateSettings" {
            n397 = case shown="\"TCP\"" w1071 {
              tunnel: w1076 -> [_ w1080 w1088]
              tunnel: w1075 -> [w1078 w1081 w1089]
              tunnel: [w1078 w1082 w1090] -> w1074
              tunnel: w1073 -> [w1077 w1083 w1091]
              tunnel: [w1077 w1083 w1086] -> w1072
              frame "False", Default {
              }
              frame "Configuration" {
                n398 = Variant To Data(error in=w1081, type="placeholder", Variant=w1080) -> (error out=w1082:errorcluster)  [unwired: 1 out]
              }
              frame "TCP" {
                w1087 = refnum<k5> refnum  # TCP
                n399 = Variant To Data(error in=w1089, type=w1087, Variant=w1088) -> (data=w1085:refnum<k5>, error out=w1090:errorcluster)
                n400 = Bundle By Name(cluster=w1091, "TCP"=w1085, "Open"=TRUE) -> (w1086:T1)
              }
            }
          }
          frame "Macro: Exit" {
            n401 = call <vilib>:"Add States to Queue using MultiLine String (no vData input).vi"("queue in"=w1095, "states in"="Quit", "error in"=w1093) -> ("error out"=w1092:errorcluster)  [unwired: 10 in, 2 out]
          }
          frame "Quit" {
          }
        }
      }
    }
  }
  n402 = Merge Errors(w12, w11) -> (w8:errorcluster)
  n403 = call <vilib>:"Clear Errors.vi"("error in (no error)"=w8) -> ("error out"=w9:errorcluster)  [unwired: 5 in, 1 out]
  n404 = Destroy User Event(user event=w10, error in=w9) -> (error out=w7:errorcluster)
  n405 = Merge Errors(w8, w7) -> (→"error out":errorcluster)
  "GIS Printer out" <- "GIS Printer in"
